vi "Checkers PvP.vi"() -> ()   [LabVIEW 2014]
uses:
  <vilib>/Utility/miscctls.llb/LVPositionTypeDef.ctl
  Game Info Global Variable.vi
  Board Layout Global Variable.vi
panel:
  out "P2 Piece 24":picture
  out "P2 Piece 23":picture
  out "P2 Piece 22":picture
  out "P2 Piece 21":picture
  out "P2 Piece 20":picture
  out "P2 Piece 19":picture
  out "P2 Piece 18":picture
  out "P2 Piece 17":picture
  out "P2 Piece 16":picture
  out "P2 Piece 15":picture
  out "P2 Piece 14":picture
  out "P2 Piece 13":picture
  out "P1 Piece 24":picture caption="P1 Piece"
  out "P1 Piece 23":picture caption="P1 Piece"
  out "P1 Piece 22":picture caption="P1 Piece"
  out "P1 Piece 21":picture caption="P1 Piece"
  out "P1 Piece 20":picture caption="P1 Piece"
  out "P1 Piece 19":picture caption="P1 Piece"
  out "P1 Piece 18":picture caption="P1 Piece"
  out "P1 Piece 17":picture caption="P1 Piece"
  out "P1 Piece 16":picture caption="P1 Piece"
  out "P1 Piece 15":picture caption="P1 Piece"
  out "P1 Piece 14":picture caption="P1 Piece"
  out "P1 Piece 13":picture caption="P1 Piece"
  out "P2 Bottom Right Marker":picture
  out "P2 Bottom Left Marker":picture
  out "P2 Top Left Marker":picture
  out "P2 Top Right Marker":picture
  out "P1 Bottom Left Marker":picture
  out "P1 Bottom Right Marker":picture
  out "P1 Top Right Marker":picture
  out "P1 Top Left Marker":picture
  in  "Save and Quit":bool
  out "Player 2 Name":string="Player 2"
  out "Player 1 Name":string="Player 1"
  out "P2 King 12":picture
  out "P2 King 11":picture
  out "P2 King 10":picture
  out "P2 King 9":picture
  out "P2 King 8":picture
  out "P2 King 7":picture
  out "P2 King 6":picture
  out "P2 King 5":picture
  out "P2 King 4":picture
  out "P2 King 3":picture
  out "P2 King 2":picture
  out "P2 King":picture
  out "P1 King 12":picture
  out "P1 King 11":picture
  out "P1 King 10":picture
  out "P1 King 9":picture
  out "P1 King 8":picture
  out "P1 King 7":picture
  out "P1 King 6":picture
  out "P1 King 5":picture
  out "P1 King 4":picture
  out "P1 King 3":picture
  out "P1 King 2":picture
  out "P1 King":picture
  out "P2 Piece Icon":picture
  out "P1 Piece Icon":picture
  out "P2 Piece 12":picture
  out "P2 Piece 11":picture
  out "P2 Piece 10":picture
  out "P2 Piece 9":picture
  out "P2 Piece 8":picture
  out "P2 Piece 7":picture
  out "P2 Piece 6":picture
  out "P2 Piece 5":picture
  out "P2 Piece 4":picture
  out "P2 Piece 3":picture
  out "P2 Piece 2":picture
  out "P1 Piece 12":picture caption="P1 Piece"
  out "P1 Piece 11":picture caption="P1 Piece"
  out "P1 Piece 10":picture caption="P1 Piece"
  out "P1 Piece 9":picture caption="P1 Piece"
  out "P1 Piece 8":picture caption="P1 Piece"
  out "P1 Piece 7":picture caption="P1 Piece"
  out "P1 Piece 6":picture caption="P1 Piece"
  out "P1 Piece 5":picture caption="P1 Piece"
  out "P1 Piece 4":picture caption="P1 Piece"
  out "P1 Piece 3":picture caption="P1 Piece"
  out "P2 Piece":picture
  out "P1 Piece 2":picture caption="P1 Piece"
  in  "TURN":bool
  out "Game String":string
  out "P2 Turn Light":bool
  out "P1 Turn Light":bool=TRUE
  out "P1 Piece":picture
  in  "stop":bool
  in  "Offer Draw":bool
  in  "Surrender":bool
  out "Player 2 Label":string="Player 1"
  out "Player 1 Label":string="Player 1"
  in  "Save":bool
  in  "Quit":bool
  # "Your Turn!"
  # "Your Turn!"
  # "678, \n56"
  # "764, \n56"
  # "512, \n56"
  # "594, \n56"
  # "637, \n99"
  # "469, \n99"
  # "553, \n99"
  # "720, \n99"
  # "355, \n141"
  # "400, \n141"
  # "512, \n140"
  # "594, \n140"
  # "678, \n140"
  # "828, \n141"
  # "873, \n141"
  # "764, \n140"
  # "828, \n184"
  # "873, \n184"
  # "355, \n184"
  # "400, \n184"
  # "469, \n183"
  # "553, \n183"
  # "637, \n183"
  # "720, \n183"
  # "355, \n225"
  # "828, \n225"
  # "873, \n225"
  # "400, \n225"
  # "764, \n224"
  # "512, \n224"
  # "595, \n224"
  # "678, \n224"
  # "828, \n267"
  # "873, \n267"
  # "355, \n267"
  # "400, \n267"
  # "469, \n266"
  # "553, \n266"
  # "720, \n266"
  # "637, \n266"
  # "355, \n309"
  # "828, \n309"
  # "400, \n309"
  # "873, \n309"
  # "678, \n308"
  # "764, \n308"
  # "512, \n308"
  # "595, \n308"
  # "355, \n351"
  # "400, \n351"
  # "873, \n351"
  # "828, \n351"
  # "553, \n350"
  # "637, \n350"
  # "720, \n350"
  # "469,\n350"
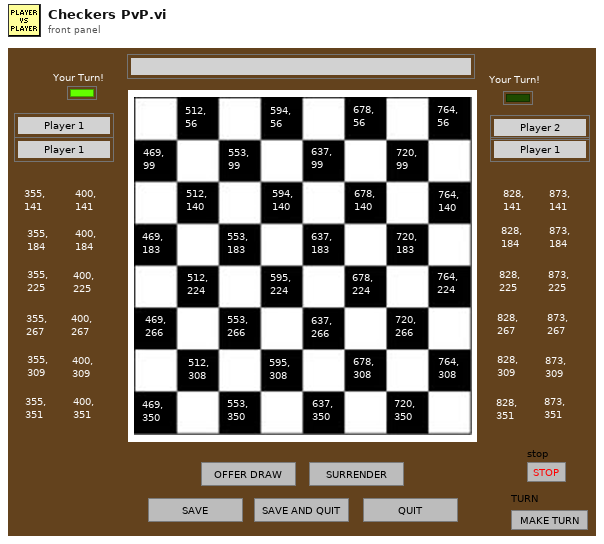
[diagram p1: front panel]
types:
  T1 = typedef "LVPositionTypeDef.ctl" = cluster{"Left":i32, "Top":i32}
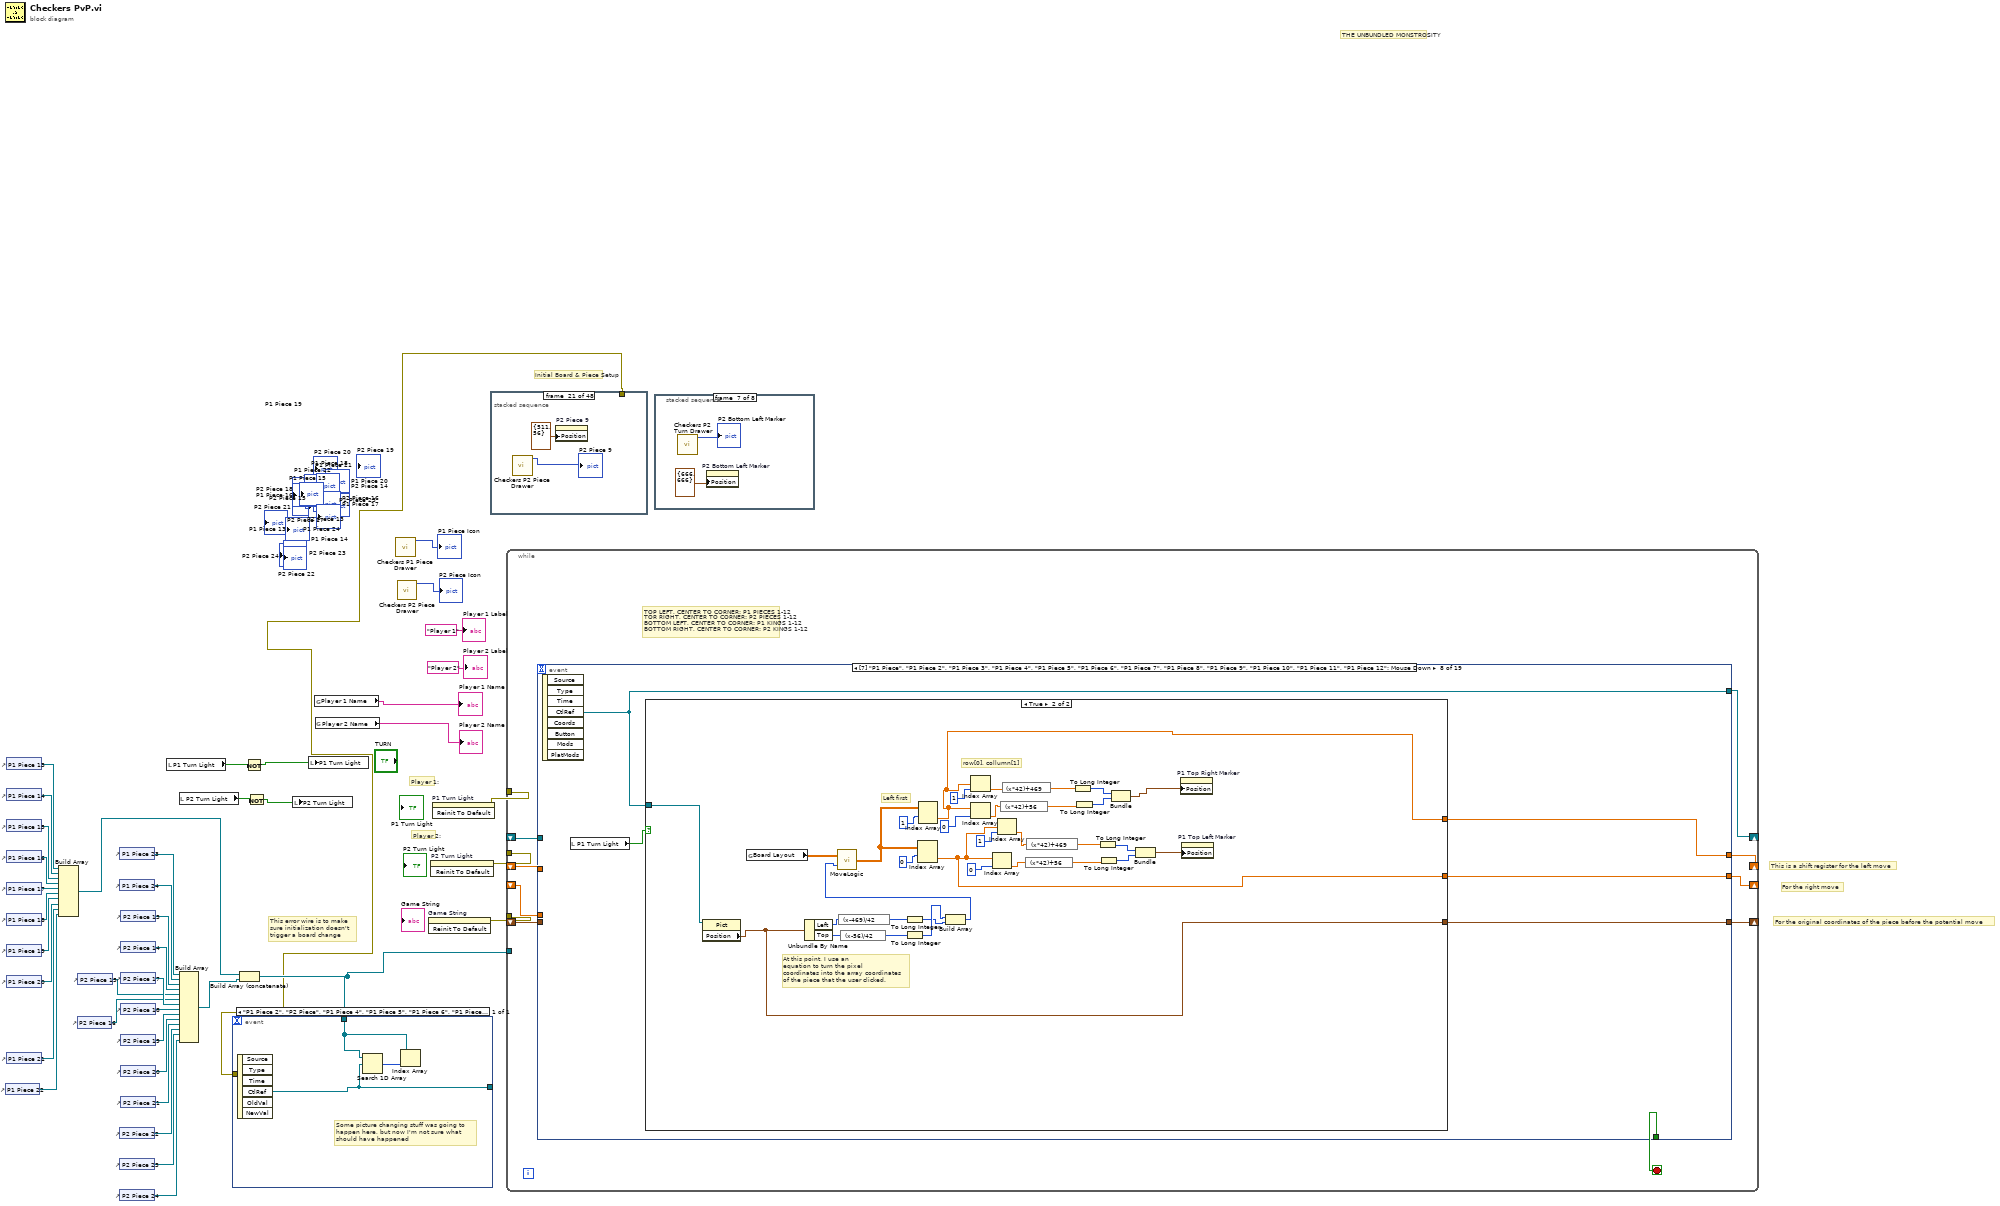
[diagram p0: block diagram]
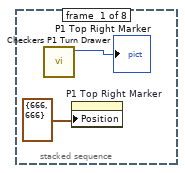
[diagram p2: hidden frame]
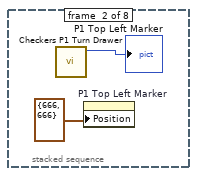
[diagram p3: hidden frame]
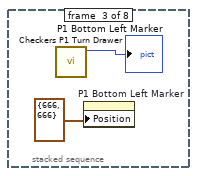
[diagram p4: hidden frame]
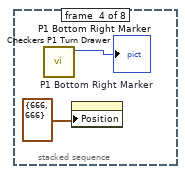
[diagram p5: hidden frame]
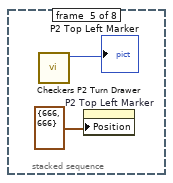
[diagram p6: hidden frame]
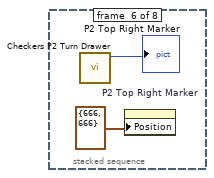
[diagram p7: hidden frame]
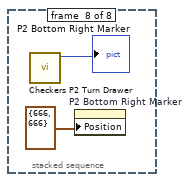
[diagram p8: hidden frame]
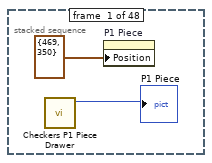
[diagram p9: hidden frame]
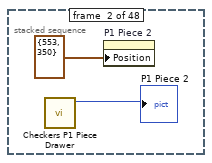
[diagram p10: hidden frame]
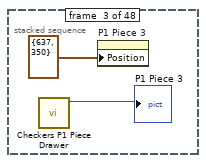
[diagram p11: hidden frame]
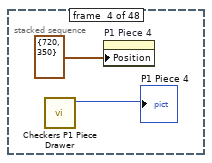
[diagram p12: hidden frame]
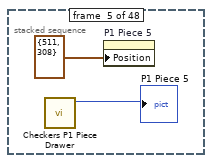
[diagram p13: hidden frame]
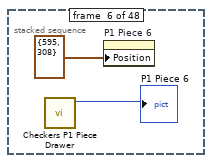
[diagram p14: hidden frame]
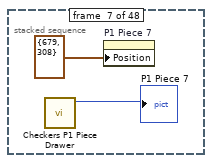
[diagram p15: hidden frame]
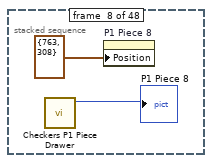
[diagram p16: hidden frame]
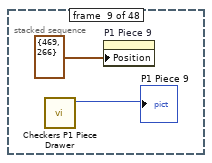
[diagram p17: hidden frame]
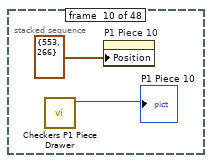
[diagram p18: hidden frame]
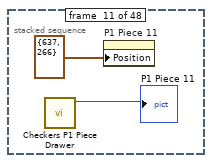
[diagram p19: hidden frame]
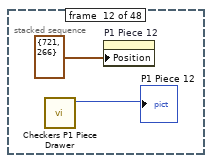
[diagram p20: hidden frame]
diagram:
  # "For the original coordinates of the piece before the potential move"
  # "For the right move"
  # "This error wire is to make \nsure initialization doesn't \ntrigger a board change"
  # "This is a shift register for the left move"
  # "THE UNBUNDLED MONSTROSITY"
  # "Initial Board & Piece Setup"
  # "Player 2:"
  # "Player 1:"
  n1 = control-ref of="P1 Piece 22"() -> (w104:refnum<vi>)
  n2 = control-ref of="P1 Piece 13"() -> (w113:refnum<vi>)
  n3 = control-ref of="P1 Piece 14"() -> (w112:refnum<vi>)
  n4 = control-ref of="P1 Piece 15"() -> (w111:refnum<vi>)
  n5 = control-ref of="P1 Piece 16"() -> (w110:refnum<vi>)
  n6 = control-ref of="P1 Piece 17"() -> (w109:refnum<vi>)
  n7 = control-ref of="P1 Piece 18"() -> (w108:refnum<vi>)
  n8 = control-ref of="P1 Piece 19"() -> (w107:refnum<vi>)
  n9 = control-ref of="P1 Piece 20"() -> (w106:refnum<vi>)
  n10 = control-ref of="P1 Piece 21"() -> (w105:refnum<vi>)
  n11 = Build Array(w113, w112, w111, w110, w109, w108, w107, w106, w105, w104) -> (w88:refnum<vi>[])
  n12 = control-ref of="P2 Piece 16"() -> (w95:refnum<vi>)
  n13 = control-ref of="P2 Piece 15"() -> (w96:refnum<vi>)
  n14 = control-ref of="P1 Piece 23"() -> (w103:refnum<vi>)
  n15 = control-ref of="P1 Piece 24"() -> (w102:refnum<vi>)
  n16 = control-ref of="P2 Piece 22"() -> (w92:refnum<vi>)
  n17 = control-ref of="P2 Piece 23"() -> (w91:refnum<vi>)
  n18 = control-ref of="P2 Piece 24"() -> (w90:refnum<vi>)
  n19 = control-ref of="P2 Piece 13"() -> (w101:refnum<vi>)
  n20 = control-ref of="P2 Piece 14"() -> (w100:refnum<vi>)
  n21 = control-ref of="P2 Piece 17"() -> (w99:refnum<vi>)
  n22 = control-ref of="P2 Piece 18"() -> (w98:refnum<vi>)
  n23 = control-ref of="P2 Piece 19"() -> (w97:refnum<vi>)
  n24 = control-ref of="P2 Piece 20"() -> (w94:refnum<vi>)
  n25 = control-ref of="P2 Piece 21"() -> (w93:refnum<vi>)
  n26 = local read "P1 Turn Light"() -> (w7:bool)
  n27 = local read "P1 Turn Light"() -> (w8:bool)
  n28 = local read "P1 Turn Light"() -> (w15:bool)
  n29 = local read "P1 Turn Light"() -> (w19:bool)
  n30 = local read "P1 Turn Light"() -> (w23:bool)
  n31 = local read "P1 Turn Light"() -> (w27:bool)
  n32 = local read "P1 Turn Light"() -> (w28:bool)
  n33 = local read "P1 Turn Light"() -> (w56:bool)
  n34 = local read "P1 Turn Light"() -> (w55:bool)
  n35 = local read "P1 Turn Light"() -> (w48:bool)
  n36 = local read "P1 Turn Light"() -> (w44:bool)
  n37 = local read "P1 Turn Light"() -> (w40:bool)
  n38 = local read "P1 Turn Light"() -> (w36:bool)
  n39 = local read "P1 Turn Light"() -> (w35:bool)
  n40 = local read "P1 Turn Light"() -> (w63:bool)
  n41 = local read "P1 Turn Light"() -> (w64:bool)
  n42 = local read "P1 Turn Light"() -> (w71:bool)
  n43 = local read "P1 Turn Light"() -> (w75:bool)
  n44 = local read "P1 Turn Light"() -> (w79:bool)
  n45 = local read "P1 Turn Light"() -> (w83:bool)
  n46 = local read "P1 Turn Light"() -> (w84:bool)
  n47 = local read "P2 Turn Light"() -> (w5:bool)
  n48 = local read "P2 Turn Light"() -> (w10:bool)
  n49 = local read "P2 Turn Light"() -> (w13:bool)
  n50 = local read "P2 Turn Light"() -> (w17:bool)
  n51 = local read "P2 Turn Light"() -> (w21:bool)
  n52 = local read "P2 Turn Light"() -> (w25:bool)
  n53 = local read "P2 Turn Light"() -> (w30:bool)
  n54 = local read "P2 Turn Light"() -> (w58:bool)
  n55 = local read "P2 Turn Light"() -> (w53:bool)
  n56 = local read "P2 Turn Light"() -> (w50:bool)
  n57 = local read "P2 Turn Light"() -> (w46:bool)
  n58 = local read "P2 Turn Light"() -> (w42:bool)
  n59 = local read "P2 Turn Light"() -> (w38:bool)
  n60 = local read "P2 Turn Light"() -> (w33:bool)
  n61 = local read "P2 Turn Light"() -> (w61:bool)
  n62 = local read "P2 Turn Light"() -> (w66:bool)
  n63 = local read "P2 Turn Light"() -> (w69:bool)
  n64 = local read "P2 Turn Light"() -> (w73:bool)
  n65 = local read "P2 Turn Light"() -> (w77:bool)
  n66 = local read "P2 Turn Light"() -> (w81:bool)
  n67 = local read "P2 Turn Light"() -> (w86:bool)
  n68 = Build Array(w103, w102, w101, w100, w96, w95, w99, w98, w97, w94, w93, w92, w91, w90) -> (w89:refnum<vi>[])
  n69 = Build Array (concatenate)(w88, w89) -> (w3:refnum<vi>[])
  n70 = Not(x=w7) -> (.not. x?=w6:bool)
  n71 = Not(x=w8) -> (.not. x?=w9:bool)
  n72 = Not(x=w15) -> (.not. x?=w14:bool)
  n73 = Not(x=w19) -> (.not. x?=w18:bool)
  n74 = Not(x=w23) -> (.not. x?=w22:bool)
  n75 = Not(x=w27) -> (.not. x?=w26:bool)
  n76 = Not(x=w28) -> (.not. x?=w29:bool)
  n77 = Not(x=w56) -> (.not. x?=w57:bool)
  n78 = Not(x=w55) -> (.not. x?=w54:bool)
  n79 = Not(x=w48) -> (.not. x?=w49:bool)
  n80 = Not(x=w44) -> (.not. x?=w45:bool)
  n81 = Not(x=w40) -> (.not. x?=w41:bool)
  n82 = Not(x=w36) -> (.not. x?=w37:bool)
  n83 = Not(x=w35) -> (.not. x?=w34:bool)
  n84 = Not(x=w63) -> (.not. x?=w62:bool)
  n85 = Not(x=w64) -> (.not. x?=w65:bool)
  n86 = Not(x=w71) -> (.not. x?=w70:bool)
  n87 = Not(x=w75) -> (.not. x?=w74:bool)
  n88 = Not(x=w79) -> (.not. x?=w78:bool)
  n89 = Not(x=w83) -> (.not. x?=w82:bool)
  n90 = Not(x=w84) -> (.not. x?=w85:bool)
  n91 = Not(x=w5) -> (.not. x?=w4:bool)
  n92 = Not(x=w10) -> (.not. x?=w11:bool)
  n93 = Not(x=w13) -> (.not. x?=w12:bool)
  n94 = Not(x=w17) -> (.not. x?=w16:bool)
  n95 = Not(x=w21) -> (.not. x?=w20:bool)
  n96 = Not(x=w25) -> (.not. x?=w24:bool)
  n97 = Not(x=w30) -> (.not. x?=w31:bool)
  n98 = Not(x=w58) -> (.not. x?=w59:bool)
  n99 = Not(x=w53) -> (.not. x?=w52:bool)
  n100 = Not(x=w50) -> (.not. x?=w51:bool)
  n101 = Not(x=w46) -> (.not. x?=w47:bool)
  n102 = Not(x=w42) -> (.not. x?=w43:bool)
  n103 = Not(x=w38) -> (.not. x?=w39:bool)
  n104 = Not(x=w33) -> (.not. x?=w32:bool)
  n105 = Not(x=w61) -> (.not. x?=w60:bool)
  n106 = Not(x=w66) -> (.not. x?=w67:bool)
  n107 = Not(x=w69) -> (.not. x?=w68:bool)
  n108 = Not(x=w73) -> (.not. x?=w72:bool)
  n109 = Not(x=w77) -> (.not. x?=w76:bool)
  n110 = Not(x=w81) -> (.not. x?=w80:bool)
  n111 = Not(x=w86) -> (.not. x?=w87:bool)
  n112 = local write "P2 Turn Light"(w4) -> ()
  n113 = local write "P2 Turn Light"(w11) -> ()
  n114 = local write "P2 Turn Light"(w12) -> ()
  n115 = local write "P2 Turn Light"(w16) -> ()
  n116 = local write "P2 Turn Light"(w20) -> ()
  n117 = local write "P2 Turn Light"(w24) -> ()
  n118 = local write "P2 Turn Light"(w31) -> ()
  n119 = local write "P2 Turn Light"(w59) -> ()
  n120 = local write "P2 Turn Light"(w52) -> ()
  n121 = local write "P2 Turn Light"(w51) -> ()
  n122 = local write "P2 Turn Light"(w47) -> ()
  n123 = local write "P2 Turn Light"(w43) -> ()
  n124 = local write "P2 Turn Light"(w39) -> ()
  n125 = local write "P2 Turn Light"(w32) -> ()
  n126 = local write "P2 Turn Light"(w60) -> ()
  n127 = local write "P2 Turn Light"(w67) -> ()
  n128 = local write "P2 Turn Light"(w68) -> ()
  n129 = local write "P2 Turn Light"(w72) -> ()
  n130 = local write "P2 Turn Light"(w76) -> ()
  n131 = local write "P2 Turn Light"(w80) -> ()
  n132 = local write "P2 Turn Light"(w87) -> ()
  n133 = local write "P1 Turn Light"(w6) -> ()
  n134 = local write "P1 Turn Light"(w9) -> ()
  n135 = local write "P1 Turn Light"(w14) -> ()
  n136 = local write "P1 Turn Light"(w18) -> ()
  n137 = local write "P1 Turn Light"(w22) -> ()
  n138 = local write "P1 Turn Light"(w26) -> ()
  n139 = local write "P1 Turn Light"(w29) -> ()
  n140 = local write "P1 Turn Light"(w57) -> ()
  n141 = local write "P1 Turn Light"(w54) -> ()
  n142 = local write "P1 Turn Light"(w49) -> ()
  n143 = local write "P1 Turn Light"(w45) -> ()
  n144 = local write "P1 Turn Light"(w41) -> ()
  n145 = local write "P1 Turn Light"(w37) -> ()
  n146 = local write "P1 Turn Light"(w34) -> ()
  n147 = local write "P1 Turn Light"(w62) -> ()
  n148 = local write "P1 Turn Light"(w65) -> ()
  n149 = local write "P1 Turn Light"(w70) -> ()
  n150 = local write "P1 Turn Light"(w74) -> ()
  n151 = local write "P1 Turn Light"(w78) -> ()
  n152 = local write "P1 Turn Light"(w82) -> ()
  n153 = local write "P1 Turn Light"(w85) -> ()
  n154 = global read "Game Info Global Variable.vi" "Player 1 Name"() -> (→"Player 1 Name":string)
  n155 = global read "Game Info Global Variable.vi" "Player 2 Name"() -> (→"Player 2 Name":string)
  n156 = call "Checkers P1 Piece Drawer.vi"() -> ("new picture"=→"P1 Piece Icon":picture)  [unwired: 11 in]
  n157 = call "Checkers P2 Piece Drawer.vi"() -> ("new picture"=→"P2 Piece Icon":picture)  [unwired: 11 in]
  n158 = invoke on="Game String" class="Str" method="Reinit To Default"() -> (error out=w117:errorcluster)  [unwired: 3 in, 2 out]
  n159 = invoke on="P2 Turn Light" class="Bool (strict)" method="Reinit To Default"() -> (error out=w119:errorcluster)  [unwired: 3 in, 2 out]
  n160 = invoke on="P1 Turn Light" class="Bool (strict)" method="Reinit To Default"() -> (error out=w118:errorcluster)  [unwired: 3 in, 2 out]
  n161 = stacked-sequence {
    tunnel: [_ _ _ _ _ _ _ _ _ _ _ _ _ _ _ _ _ _ _ _ _ _ _ _ _ _ _ _ _ _ _ _ _ _ _ _ _ _ _ _ _ _ _ _ _ _ _ w216] -> w1
    frame #0 {
      n162 = call "Checkers P1 Piece Drawer.vi"() -> ("new picture"=→"P1 Piece":picture)  [unwired: 11 in]
      n163 = property on="P1 Piece" class="Pict"("Position"=T1 {"Left"=469, "Top"=350}) -> ()  [unwired: 2 in, 2 out]
    }
    frame #1 {
      n164 = call "Checkers P1 Piece Drawer.vi"() -> ("new picture"=→"P1 Piece 2":picture)  [unwired: 11 in]
      n165 = property on="P1 Piece 2" class="Pict"("Position"=T1 {"Left"=553, "Top"=350}) -> ()  [unwired: 2 in, 2 out]
    }
    frame #2 {
      n166 = call "Checkers P1 Piece Drawer.vi"() -> ("new picture"=→"P1 Piece 3":picture)  [unwired: 11 in]
      n167 = property on="P1 Piece 3" class="Pict"("Position"=T1 {"Left"=637, "Top"=350}) -> ()  [unwired: 2 in, 2 out]
    }
    frame #3 {
      n168 = call "Checkers P1 Piece Drawer.vi"() -> ("new picture"=→"P1 Piece 4":picture)  [unwired: 11 in]
      n169 = property on="P1 Piece 4" class="Pict"("Position"=T1 {"Left"=720, "Top"=350}) -> ()  [unwired: 2 in, 2 out]
    }
    frame #4 {
      n170 = call "Checkers P1 Piece Drawer.vi"() -> ("new picture"=→"P1 Piece 5":picture)  [unwired: 11 in]
      n171 = property on="P1 Piece 5" class="Pict"("Position"=T1 {"Left"=511, "Top"=308}) -> ()  [unwired: 2 in, 2 out]
    }
    frame #5 {
      n172 = call "Checkers P1 Piece Drawer.vi"() -> ("new picture"=→"P1 Piece 6":picture)  [unwired: 11 in]
      n173 = property on="P1 Piece 6" class="Pict"("Position"=T1 {"Left"=595, "Top"=308}) -> ()  [unwired: 2 in, 2 out]
    }
    frame #6 {
      n174 = call "Checkers P1 Piece Drawer.vi"() -> ("new picture"=→"P1 Piece 7":picture)  [unwired: 11 in]
      n175 = property on="P1 Piece 7" class="Pict"("Position"=T1 {"Left"=679, "Top"=308}) -> ()  [unwired: 2 in, 2 out]
    }
    frame #7 {
      n176 = call "Checkers P1 Piece Drawer.vi"() -> ("new picture"=→"P1 Piece 8":picture)  [unwired: 11 in]
      n177 = property on="P1 Piece 8" class="Pict"("Position"=T1 {"Left"=763, "Top"=308}) -> ()  [unwired: 2 in, 2 out]
    }
    frame #8 {
      n178 = call "Checkers P1 Piece Drawer.vi"() -> ("new picture"=→"P1 Piece 9":picture)  [unwired: 11 in]
      n179 = property on="P1 Piece 9" class="Pict"("Position"=T1 {"Left"=469, "Top"=266}) -> ()  [unwired: 2 in, 2 out]
    }
    frame #9 {
      n180 = call "Checkers P1 Piece Drawer.vi"() -> ("new picture"=→"P1 Piece 10":picture)  [unwired: 11 in]
      n181 = property on="P1 Piece 10" class="Pict"("Position"=T1 {"Left"=553, "Top"=266}) -> ()  [unwired: 2 in, 2 out]
    }
    frame #10 {
      n182 = call "Checkers P1 Piece Drawer.vi"() -> ("new picture"=→"P1 Piece 11":picture)  [unwired: 11 in]
      n183 = property on="P1 Piece 11" class="Pict"("Position"=T1 {"Left"=637, "Top"=266}) -> ()  [unwired: 2 in, 2 out]
    }
    frame #11 {
      n184 = call "Checkers P1 Piece Drawer.vi"() -> ("new picture"=→"P1 Piece 12":picture)  [unwired: 11 in]
      n185 = property on="P1 Piece 12" class="Pict"("Position"=T1 {"Left"=721, "Top"=266}) -> ()  [unwired: 2 in, 2 out]
    }
    frame #12 {
      n186 = call "Checkers P2 Piece Drawer.vi"() -> ("new picture"=→"P2 Piece":picture)  [unwired: 11 in]
      n187 = property on="P2 Piece" class="Pict"("Position"=T1 {"Left"=511, "Top"=140}) -> ()  [unwired: 2 in, 2 out]
    }
    frame #13 {
      n188 = call "Checkers P2 Piece Drawer.vi"() -> ("new picture"=→"P2 Piece 2":picture)  [unwired: 11 in]
      n189 = property on="P2 Piece 2" class="Pict"("Position"=T1 {"Left"=595, "Top"=140}) -> ()  [unwired: 2 in, 2 out]
    }
    frame #14 {
      n190 = call "Checkers P2 Piece Drawer.vi"() -> ("new picture"=→"P2 Piece 3":picture)  [unwired: 11 in]
      n191 = property on="P2 Piece 3" class="Pict"("Position"=T1 {"Left"=679, "Top"=140}) -> ()  [unwired: 2 in, 2 out]
    }
    frame #15 {
      n192 = call "Checkers P2 Piece Drawer.vi"() -> ("new picture"=→"P2 Piece 4":picture)  [unwired: 11 in]
      n193 = property on="P2 Piece 4" class="Pict"("Position"=T1 {"Left"=763, "Top"=140}) -> ()  [unwired: 2 in, 2 out]
    }
    frame #16 {
      n194 = call "Checkers P2 Piece Drawer.vi"() -> ("new picture"=→"P2 Piece 5":picture)  [unwired: 11 in]
      n195 = property on="P2 Piece 5" class="Pict"("Position"=T1 {"Left"=469, "Top"=98}) -> ()  [unwired: 2 in, 2 out]
    }
    frame #17 {
      n196 = call "Checkers P2 Piece Drawer.vi"() -> ("new picture"=→"P2 Piece 6":picture)  [unwired: 11 in]
      n197 = property on="P2 Piece 6" class="Pict"("Position"=T1 {"Left"=553, "Top"=98}) -> ()  [unwired: 2 in, 2 out]
    }
    frame #18 {
      n198 = call "Checkers P2 Piece Drawer.vi"() -> ("new picture"=→"P2 Piece 7":picture)  [unwired: 11 in]
      n199 = property on="P2 Piece 7" class="Pict"("Position"=T1 {"Left"=637, "Top"=98}) -> ()  [unwired: 2 in, 2 out]
    }
    frame #19 {
      n200 = call "Checkers P2 Piece Drawer.vi"() -> ("new picture"=→"P2 Piece 8":picture)  [unwired: 11 in]
      n201 = property on="P2 Piece 8" class="Pict"("Position"=T1 {"Left"=721, "Top"=98}) -> ()  [unwired: 2 in, 2 out]
    }
    frame #20 {
      n202 = call "Checkers P2 Piece Drawer.vi"() -> ("new picture"=→"P2 Piece 9":picture)  [unwired: 11 in]
      n203 = property on="P2 Piece 9" class="Pict"("Position"=T1 {"Left"=511, "Top"=56}) -> ()  [unwired: 2 in, 2 out]
    }
    frame #21 {
      n204 = call "Checkers P2 Piece Drawer.vi"() -> ("new picture"=→"P2 Piece 10":picture)  [unwired: 11 in]
      n205 = property on="P2 Piece 10" class="Pict"("Position"=T1 {"Left"=595, "Top"=56}) -> ()  [unwired: 2 in, 2 out]
    }
    frame #22 {
      n206 = call "Checkers P2 Piece Drawer.vi"() -> ("new picture"=→"P2 Piece 11":picture)  [unwired: 11 in]
      n207 = property on="P2 Piece 11" class="Pict"("Position"=T1 {"Left"=679, "Top"=56}) -> ()  [unwired: 2 in, 2 out]
    }
    frame #23 {
      n208 = call "Checkers P2 Piece Drawer.vi"() -> ("new picture"=→"P2 Piece 12":picture)  [unwired: 11 in]
      n209 = property on="P2 Piece 12" class="Pict"("Position"=T1 {"Left"=763, "Top"=56}) -> ()  [unwired: 2 in, 2 out]
    }
    frame #24 {
      n210 = call "Checkers P1 King Drawer.vi"() -> ("new picture"=→"P1 King":picture)  [unwired: 11 in]
      n211 = property on="P1 King" class="Pict"("Position"=T1 {"Left"=666, "Top"=666}) -> ()  [unwired: 2 in, 2 out]
    }
    frame #25 {
      n212 = call "Checkers P1 King Drawer.vi"() -> ("new picture"=→"P1 King 2":picture)  [unwired: 11 in]
      n213 = property on="P1 King 2" class="Pict"("Position"=T1 {"Left"=666, "Top"=666}) -> ()  [unwired: 2 in, 2 out]
    }
    frame #26 {
      n214 = call "Checkers P1 King Drawer.vi"() -> ("new picture"=→"P1 King 3":picture)  [unwired: 11 in]
      n215 = property on="P1 King 3" class="Pict"("Position"=T1 {"Left"=666, "Top"=666}) -> ()  [unwired: 2 in, 2 out]
    }
    frame #27 {
      n216 = call "Checkers P1 King Drawer.vi"() -> ("new picture"=→"P1 King 4":picture)  [unwired: 11 in]
      n217 = property on="P1 King 4" class="Pict"("Position"=T1 {"Left"=666, "Top"=666}) -> ()  [unwired: 2 in, 2 out]
    }
    frame #28 {
      n218 = call "Checkers P1 King Drawer.vi"() -> ("new picture"=→"P1 King 5":picture)  [unwired: 11 in]
      n219 = property on="P1 King 5" class="Pict"("Position"=T1 {"Left"=666, "Top"=666}) -> ()  [unwired: 2 in, 2 out]
    }
    frame #29 {
      n220 = call "Checkers P1 King Drawer.vi"() -> ("new picture"=→"P1 King 6":picture)  [unwired: 11 in]
      n221 = property on="P1 King 6" class="Pict"("Position"=T1 {"Left"=666, "Top"=666}) -> ()  [unwired: 2 in, 2 out]
    }
    frame #30 {
      n222 = call "Checkers P1 King Drawer.vi"() -> ("new picture"=→"P1 King 7":picture)  [unwired: 11 in]
      n223 = property on="P1 King 7" class="Pict"("Position"=T1 {"Left"=666, "Top"=666}) -> ()  [unwired: 2 in, 2 out]
    }
    frame #31 {
      n224 = call "Checkers P1 King Drawer.vi"() -> ("new picture"=→"P1 King 8":picture)  [unwired: 11 in]
      n225 = property on="P1 King 8" class="Pict"("Position"=T1 {"Left"=666, "Top"=666}) -> ()  [unwired: 2 in, 2 out]
    }
    frame #32 {
      n226 = call "Checkers P1 King Drawer.vi"() -> ("new picture"=→"P1 King 9":picture)  [unwired: 11 in]
      n227 = property on="P1 King 9" class="Pict"("Position"=T1 {"Left"=666, "Top"=666}) -> ()  [unwired: 2 in, 2 out]
    }
    frame #33 {
      n228 = call "Checkers P1 King Drawer.vi"() -> ("new picture"=→"P1 King 10":picture)  [unwired: 11 in]
      n229 = property on="P1 King 10" class="Pict"("Position"=T1 {"Left"=666, "Top"=666}) -> ()  [unwired: 2 in, 2 out]
    }
    frame #34 {
      n230 = call "Checkers P1 King Drawer.vi"() -> ("new picture"=→"P1 King 11":picture)  [unwired: 11 in]
      n231 = property on="P1 King 11" class="Pict"("Position"=T1 {"Left"=666, "Top"=666}) -> ()  [unwired: 2 in, 2 out]
    }
    frame #35 {
      n232 = call "Checkers P1 King Drawer.vi"() -> ("new picture"=→"P1 King 12":picture)  [unwired: 11 in]
      n233 = property on="P1 King 12" class="Pict"("Position"=T1 {"Left"=666, "Top"=666}) -> ()  [unwired: 2 in, 2 out]
    }
    frame #36 {
      n234 = call "Checkers P2 King Drawer.vi"() -> ("new picture"=→"P2 King":picture)  [unwired: 11 in]
      n235 = property on="P2 King" class="Pict"("Position"=T1 {"Left"=666, "Top"=666}) -> ()  [unwired: 2 in, 2 out]
    }
    frame #37 {
      n236 = call "Checkers P2 King Drawer.vi"() -> ("new picture"=→"P2 King 2":picture)  [unwired: 11 in]
      n237 = property on="P2 King 2" class="Pict"("Position"=T1 {"Left"=666, "Top"=666}) -> ()  [unwired: 2 in, 2 out]
    }
    frame #38 {
      n238 = call "Checkers P2 King Drawer.vi"() -> ("new picture"=→"P2 King 3":picture)  [unwired: 11 in]
      n239 = property on="P2 King 3" class="Pict"("Position"=T1 {"Left"=666, "Top"=666}) -> ()  [unwired: 2 in, 2 out]
    }
    frame #39 {
      n240 = call "Checkers P2 King Drawer.vi"() -> ("new picture"=→"P2 King 4":picture)  [unwired: 11 in]
      n241 = property on="P2 King 4" class="Pict"("Position"=T1 {"Left"=666, "Top"=666}) -> ()  [unwired: 2 in, 2 out]
    }
    frame #40 {
      n242 = call "Checkers P2 King Drawer.vi"() -> ("new picture"=→"P2 King 5":picture)  [unwired: 11 in]
      n243 = property on="P2 King 5" class="Pict"("Position"=T1 {"Left"=666, "Top"=666}) -> ()  [unwired: 2 in, 2 out]
    }
    frame #41 {
      n244 = call "Checkers P2 King Drawer.vi"() -> ("new picture"=→"P2 King 6":picture)  [unwired: 11 in]
      n245 = property on="P2 King 6" class="Pict"("Position"=T1 {"Left"=666, "Top"=666}) -> ()  [unwired: 2 in, 2 out]
    }
    frame #42 {
      n246 = call "Checkers P2 King Drawer.vi"() -> ("new picture"=→"P2 King 7":picture)  [unwired: 11 in]
      n247 = property on="P2 King 7" class="Pict"("Position"=T1 {"Left"=666, "Top"=666}) -> ()  [unwired: 2 in, 2 out]
    }
    frame #43 {
      n248 = call "Checkers P2 King Drawer.vi"() -> ("new picture"=→"P2 King 8":picture)  [unwired: 11 in]
      n249 = property on="P2 King 8" class="Pict"("Position"=T1 {"Left"=666, "Top"=666}) -> ()  [unwired: 2 in, 2 out]
    }
    frame #44 {
      n250 = call "Checkers P2 King Drawer.vi"() -> ("new picture"=→"P2 King 9":picture)  [unwired: 11 in]
      n251 = property on="P2 King 9" class="Pict"("Position"=T1 {"Left"=666, "Top"=666}) -> ()  [unwired: 2 in, 2 out]
    }
    frame #45 {
      n252 = call "Checkers P2 King Drawer.vi"() -> ("new picture"=→"P2 King 10":picture)  [unwired: 11 in]
      n253 = property on="P2 King 10" class="Pict"("Position"=T1 {"Left"=666, "Top"=666}) -> ()  [unwired: 2 in, 2 out]
    }
    frame #46 {
      n254 = call "Checkers P2 King Drawer.vi"() -> ("new picture"=→"P2 King 11":picture)  [unwired: 11 in]
      n255 = property on="P2 King 11" class="Pict"("Position"=T1 {"Left"=666, "Top"=666}) -> ()  [unwired: 2 in, 2 out]
    }
    frame #47 {
      n256 = call "Checkers P2 King Drawer.vi"() -> ("new picture"=→"P2 King 12":picture)  [unwired: 11 in]
      n257 = property on="P2 King 12" class="Pict"("Position"=T1 {"Left"=666, "Top"=666}) -> (error out=w216:errorcluster)  [unwired: 2 in, 1 out]
    }
  }
  n258 = event shown="[0] \"P1 Piece 2\", \"P2 Piece\", \"P1 Piece 4\", \"P1 Piece 5\", \"P1 Piece 6\", \"P1 Piece 7\", \"P1 Piece 8\", \"P1 Piece 9\", \"P1 Piece 10\", \"P1 Piece 11\", \"P1 Piece 12\", \"P2 Piece 2\", \"P2 Piece 3\", \"P2 Piece 4\", \"P2 Piece 6\", \"P2 Piece 7\", \"P2 Piece 8\", \"P2 Piece 9\", \"P2 Piece 10\", \"P2 Piece 11\", \"P2 Piece 12\": Value Change" {
    selector: _ -> [_]
    dyn-events: _ -> [_]
    timeout: _ -> [_]
    tunnel: [w221] -> _
    tunnel: w3 -> [w220]
    tunnel: w1 -> [_]
    event "P1 Piece 2", "P2 Piece", "P1 Piece 4", "P1 Piece 5", "P1 Piece 6", "P1 Piece 7", "P1 Piece 8", "P1 Piece 9", "P1 Piece 10", "P1 Piece 11", "P1 Piece 12", "P2 Piece 2", "P2 Piece 3", "P2 Piece 4", "P2 Piece 6", "P2 Piece 7", "P2 Piece 8", "P2 Piece 9", "P2 Piece 10", "P2 Piece 11", "P2 Piece 12": Value Change {
      # "Some picture changing stuff was going to \nhappen here, but now I'm not sure what \nshould have happened"
      n259 = event-data() -> ("CtlRef"=w221:refnum<vi>)  [unwired: 1 in, 5 out]
      n260 = Search 1D Array(1D array=w220, element=w221) -> (index of element=w219:i32)  [unwired: 1 in]
      n261 = Index Array(array=w220, index=w219) -> ()  [unwired: 1 out]
    }
  }
  n262 = while {
    tunnel: w119 -> [_]
    tunnel: w118 -> [_]
    tunnel: w117 -> [_]
    tunnel: w3 -> [_]
    shift-right: [w229] -> _
    shift-left: _ -> [w228]
    shift-right: [w227] -> _
    shift-left: _ -> [w222]
    shift-right: [w226] -> _
    shift-left: _ -> [w225]
    shift-right: [w224] -> _
    shift-left: _ -> [w223]
    stop <- w230 stop-if-true
    # "TOP LEFT, CENTER TO CORNER: P1 PIECES 1-12\nTOR RIGHT, CENTER TO CORNER: P2 PIECES 1-12\nBOTTOM LEFT, CENTER TO CORNER: P1 KINGS 1-12\nBOTTOM RIGHT, CENTER TO CORNER: P2 KINGS 1-12"
    n263 = event shown="[7] \"P1 Piece\", \"P1 Piece 2\", \"P1 Piece 3\", \"P1 Piece 4\", \"P1 Piece 5\", \"P1 Piece 6\", \"P1 Piece 7\", \"P1 Piece 8\", \"P1 Piece 9\", \"P1 Piece 10\", \"P1 Piece 11\", \"P1 Piece 12\": Mouse Down" {
      selector: _ -> [_ _ _ _ _ _ _ _ _ _ _ _ _ _ _ _ _ _ _]
      dyn-events: _ -> [_ _ _ _ _ _ _ _ _ _ _ _ _ _ _ _ _ _ _]
      timeout: _ -> [_ _ _ _ _ _ _ _ _ _ _ _ _ _ _ _ _ _ _]
      tunnel: [_ "stop" _ _ _ _ _ _ _ _ _ _ _ _ _ _ _ _ _] -> w230
      tunnel: [_ _ _ _ _ _ _ w605 w640 w675 w710 _ _ _ _ _ _ _ _] -> w229
      tunnel: w228 -> [_ _ _ _ _ _ _ _ _ _ _ w755 w766 w777 w788 w799 w814 w849 w940]
      tunnel: [_ _ _ _ _ _ _ w604 _ _ _ _ _ _ _ _ _ _ _] -> w227
      tunnel: [_ _ _ _ _ _ _ w603 _ _ _ _ _ _ _ _ _ _ _] -> w226
      tunnel: w225 -> [_ _ _ _ _ _ _ _ _ _ _ w748 _ _ _ _ _ _ _]
      tunnel: [_ _ _ _ _ _ _ w602 _ _ _ _ _ _ _ _ _ _ _] -> w224
      tunnel: w223 -> [_ _ _ _ _ _ _ _ _ _ _ w747 _ _ _ _ w801 _ _]
      tunnel: w222 -> [_ _ _ _ _ _ _ _ _ _ _ _ _ _ _ _ w800 _ _]
      event Timeout {
        n264 = event-data() -> ()  [unwired: 1 in, 3 out]
      }
      event "stop": Value Change {
        n265 = event-data() -> ()  [unwired: 1 in, 6 out]
      }
      event "Offer Draw": Value Change {
        n266 = event-data() -> ()  [unwired: 1 in, 6 out]
        n267 = local read "P1 Turn Light"() -> (w232:bool)
        n268 = case shown="False" w232 {
          frame False {
            n269 = local read "Player 2 Name"() -> (w236:string)
            n270 = Format Into String(format string="%s offers a stalemate. Do you accept?", w236) -> (resulting string=w234:string)  [unwired: 2 in, 1 out]
            n271 = Two Button Dialog(message=w234, 1:"Decline" ("F button name (\"Cancel\")"), 2:"Accept" ("T button name (\"OK\")")) -> (T button?=w233:bool)
            n272 = case shown="True" w233 {
              frame False {
                # "Stalemate offer rejected. Do nothing."
              }
              frame True {
                w239 = "GAME OVER. It's a draw." ("format string")
                n273 = local write "Game String"(w239) -> ()
                n274 = Two Button Dialog(message=w239, 1:"Main Menu" ("F button name (\"Cancel\")"), 2:"New Game" ("T button name (\"OK\")")) -> (T button?=w242:bool)
                n275 = case shown="False" w242 {
                  frame False {
                    n276 = vi-ref "Checkers Main Menu.vi"() -> (w249:refnum<vi>)
                    n277 = invoke class="VI" method="Run VI"(reference=w249, "Wait until done"=FALSE ("Wait Until Done")) -> (reference out=w248:refnum<vi>, error out=w247:errorcluster)  [unwired: 3 in, 3 out]
                    n278 = invoke class="VI" method="FP.Open"(reference=w248, error in=w247, "Activate"=TRUE ("Activate?")) -> (error out=w246:errorcluster)  [unwired: 2 in, 4 out]
                    n279 = vi-ref "Checkers PvP.vi"() -> (w245:refnum<vi>)
                    n280 = invoke class="VI" method="Abort VI"(reference=w245, error in=w246) -> ()  [unwired: 1 in, 3 out]
                  }
                  frame True {
                    n281 = vi-ref "Checkers New Game.vi"() -> (w256:refnum<vi>)
                    n282 = invoke class="VI" method="Run VI"(reference=w256, "Wait until done"=FALSE ("Wait Until Done")) -> (reference out=w255:refnum<vi>, error out=w254:errorcluster)  [unwired: 3 in, 3 out]
                    n283 = invoke class="VI" method="FP.Open"(reference=w255, error in=w254, "Activate"=TRUE ("Activate?")) -> (error out=w253:errorcluster)  [unwired: 2 in, 4 out]
                    n284 = vi-ref "Checkers PvP.vi"() -> (w252:refnum<vi>)
                    n285 = invoke class="VI" method="Abort VI"(reference=w252, error in=w253) -> ()  [unwired: 1 in, 3 out]
                  }
                }
              }
            }
          }
          frame True {
            n286 = local read "Player 1 Name"() -> (w260:string)
            n287 = Format Into String(format string="%s offers a stalemate. Do you accept?", w260) -> (resulting string=w258:string)  [unwired: 2 in, 1 out]
            n288 = Two Button Dialog(message=w258, 1:"Decline" ("F button name (\"Cancel\")"), 2:"Accept" ("T button name (\"OK\")")) -> (T button?=w257:bool)
            n289 = case shown="True" w257 {
              frame False {
                # "Stalemate offer was rejected. Do nothing."
              }
              frame True {
                w263 = "GAME OVER. Stalemate." ("format string")
                n290 = local write "Game String"(w263) -> ()
                n291 = Two Button Dialog(message=w263, 1:"Main Menu" ("F button name (\"Cancel\")"), 2:"New Game" ("T button name (\"OK\")")) -> (T button?=w266:bool)
                n292 = case shown="False" w266 {
                  frame False {
                    n293 = vi-ref "Checkers Main Menu.vi"() -> (w273:refnum<vi>)
                    n294 = invoke class="VI" method="Run VI"(reference=w273, "Wait until done"=FALSE ("Wait Until Done")) -> (reference out=w272:refnum<vi>, error out=w271:errorcluster)  [unwired: 3 in, 3 out]
                    n295 = invoke class="VI" method="FP.Open"(reference=w272, error in=w271, "Activate"=TRUE ("Activate?")) -> (error out=w270:errorcluster)  [unwired: 2 in, 4 out]
                    n296 = vi-ref "Checkers PvP.vi"() -> (w269:refnum<vi>)
                    n297 = invoke class="VI" method="Abort VI"(reference=w269, error in=w270) -> ()  [unwired: 1 in, 3 out]
                  }
                  frame True {
                    n298 = vi-ref "Checkers New Game.vi"() -> (w280:refnum<vi>)
                    n299 = invoke class="VI" method="Run VI"(reference=w280, "Wait until done"=FALSE ("Wait Until Done")) -> (reference out=w279:refnum<vi>, error out=w278:errorcluster)  [unwired: 3 in, 3 out]
                    n300 = invoke class="VI" method="FP.Open"(reference=w279, error in=w278, "Activate"=TRUE ("Activate?")) -> (error out=w277:errorcluster)  [unwired: 2 in, 4 out]
                    n301 = vi-ref "Checkers PvP.vi"() -> (w276:refnum<vi>)
                    n302 = invoke class="VI" method="Abort VI"(reference=w276, error in=w277) -> ()  [unwired: 1 in, 3 out]
                  }
                }
              }
            }
          }
        }
      }
      event "Surrender": Value Change {
        n303 = event-data() -> ()  [unwired: 1 in, 6 out]
        n304 = Two Button Dialog(message="Are you sure you want to surrender?", 1:"No" ("F button name (\"Cancel\")"), 2:"Yes" ("T button name (\"OK\")")) -> (T button?=w281:bool)
        n305 = case shown="True" w281 {
          frame False {
            # "Player changed mind, didn't surrender. Do nothing."
          }
          frame True {
            n306 = local read "P1 Turn Light"() -> (w285:bool)
            n307 = case shown="True" w285 {
              frame False {
                n308 = local read "Player 1 Name"() -> (w286:string)
                n309 = Format Into String(format string="GAME OVER. %s WINS!", w286) -> (resulting string=w290:string)  [unwired: 2 in, 1 out]
                n310 = local write "Game String"(w290) -> ()
                n311 = Two Button Dialog(message=w290, 1:"Main Menu" ("F button name (\"Cancel\")"), 2:"New Game" ("T button name (\"OK\")")) -> (T button?=w287:bool)
                n312 = case shown="True" w287 {
                  frame False {
                    n313 = vi-ref "Checkers Main Menu.vi"() -> (w298:refnum<vi>)
                    n314 = invoke class="VI" method="Run VI"(reference=w298, "Wait until done"=FALSE ("Wait Until Done")) -> (reference out=w297:refnum<vi>, error out=w296:errorcluster)  [unwired: 3 in, 3 out]
                    n315 = invoke class="VI" method="FP.Open"(reference=w297, error in=w296, "Activate"=TRUE ("Activate?")) -> (error out=w295:errorcluster)  [unwired: 2 in, 4 out]
                    n316 = vi-ref "Checkers PvP.vi"() -> (w294:refnum<vi>)
                    n317 = invoke class="VI" method="Abort VI"(reference=w294, error in=w295) -> ()  [unwired: 1 in, 3 out]
                  }
                  frame True {
                    n318 = vi-ref "Checkers New Game.vi"() -> (w308:refnum<vi>)
                    n319 = vi-ref "Checkers Gymnopedie Music Player.vi"() -> (w299:refnum<vi>)
                    n320 = invoke class="VI" method="Run VI"(reference=w299, "Wait until done"=FALSE ("Wait Until Done")) -> ()  [unwired: 3 in, 5 out]
                    n321 = invoke class="VI" method="Run VI"(reference=w308, "Wait until done"=FALSE ("Wait Until Done")) -> (reference out=w307:refnum<vi>, error out=w306:errorcluster)  [unwired: 3 in, 3 out]
                    n322 = vi-ref "Checkers Palladio Music Player.vi"() -> (w301:refnum<vi>)
                    n323 = invoke class="VI" method="FP.Open"(reference=w307, error in=w306, "Activate"=TRUE ("Activate?")) -> (error out=w305:errorcluster)  [unwired: 2 in, 4 out]
                    n324 = vi-ref "Checkers PvP.vi"() -> (w304:refnum<vi>)
                    n325 = invoke class="VI" method="Abort VI"(reference=w301) -> ()  [unwired: 2 in, 3 out]
                    n326 = invoke class="VI" method="Abort VI"(reference=w304, error in=w305) -> ()  [unwired: 1 in, 3 out]
                  }
                }
              }
              frame True {
                n327 = local read "Player 2 Name"() -> (w309:string)
                n328 = Format Into String(format string="GAME OVER. %s WINS!", w309) -> (resulting string=w313:string)  [unwired: 2 in, 1 out]
                n329 = local write "Game String"(w313) -> ()
                n330 = Two Button Dialog(message=w313, 1:"Main Menu" ("F button name (\"Cancel\")"), 2:"New Game" ("T button name (\"OK\")")) -> (T button?=w310:bool)
                n331 = case shown="True" w310 {
                  frame False {
                    n332 = vi-ref "Checkers Main Menu.vi"() -> (w321:refnum<vi>)
                    n333 = invoke class="VI" method="Run VI"(reference=w321, "Wait until done"=FALSE ("Wait Until Done")) -> (reference out=w320:refnum<vi>, error out=w319:errorcluster)  [unwired: 3 in, 3 out]
                    n334 = invoke class="VI" method="FP.Open"(reference=w320, error in=w319, "Activate"=TRUE ("Activate?")) -> (error out=w318:errorcluster)  [unwired: 2 in, 4 out]
                    n335 = vi-ref "Checkers PvP.vi"() -> (w317:refnum<vi>)
                    n336 = invoke class="VI" method="Abort VI"(reference=w317, error in=w318) -> ()  [unwired: 1 in, 3 out]
                  }
                  frame True {
                    n337 = vi-ref "Checkers New Game.vi"() -> (w331:refnum<vi>)
                    n338 = vi-ref "Checkers Gymnopedie Music Player.vi"() -> (w322:refnum<vi>)
                    n339 = invoke class="VI" method="Run VI"(reference=w331, "Wait until done"=FALSE ("Wait Until Done")) -> (reference out=w330:refnum<vi>, error out=w329:errorcluster)  [unwired: 3 in, 3 out]
                    n340 = invoke class="VI" method="Run VI"(reference=w322, "Wait until done"=FALSE ("Wait Until Done")) -> ()  [unwired: 3 in, 5 out]
                    n341 = vi-ref "Checkers Palladio Music Player.vi"() -> (w324:refnum<vi>)
                    n342 = invoke class="VI" method="FP.Open"(reference=w330, error in=w329, "Activate"=TRUE ("Activate?")) -> (error out=w328:errorcluster)  [unwired: 2 in, 4 out]
                    n343 = vi-ref "Checkers PvP.vi"() -> (w327:refnum<vi>)
                    n344 = invoke class="VI" method="Abort VI"(reference=w324) -> ()  [unwired: 2 in, 3 out]
                    n345 = invoke class="VI" method="Abort VI"(reference=w327, error in=w328) -> ()  [unwired: 1 in, 3 out]
                  }
                }
              }
            }
          }
        }
      }
      event "Save": Value Change {
        n346 = event-data() -> ()  [unwired: 1 in, 6 out]
        n347 = global read "Game Info Global Variable.vi" "P1 King Text Green Color"() -> (w391:i32)
        n348 = global read "Game Info Global Variable.vi" "P2 King Text Green Color"() -> (w385:i32)
        n349 = global read "Game Info Global Variable.vi" "P1 King Text Blue Color"() -> (w390:i32)
        n350 = global read "Game Info Global Variable.vi" "P2 King Text Blue Color"() -> (w384:i32)
        n351 = global read "Game Info Global Variable.vi" "P1 King Text Red Color"() -> (w392:i32)
        n352 = global read "Game Info Global Variable.vi" "P2 King Text Red Color"() -> (w386:i32)
        n353 = global read "Game Info Global Variable.vi" "P1 Green Color"() -> (w394:i32)
        n354 = global read "Game Info Global Variable.vi" "P2 Green Color"() -> (w388:i32)
        n355 = local read "Player 1 Name"() -> (w398:string)
        n356 = local read "Player 2 Name"() -> (w397:string)
        n357 = global read "Game Info Global Variable.vi" "P1 Red Color"() -> (w395:i32)
        n358 = global read "Game Info Global Variable.vi" "P1 Blue Color"() -> (w393:i32)
        n359 = global read "Game Info Global Variable.vi" "P2 Blue Color"() -> (w387:i32)
        n360 = global read "Game Info Global Variable.vi" "P2 Red Color"() -> (w389:i32)
        n361 = Format Into String(w398, w397, w395, w394, w393, w392, w391, w390, w389, w388, w387, w386, w385, w384) -> (resulting string=w396:refnum<file>)  [unwired: 3 in, 1 out]
        n362 = stacked-sequence {
          tunnel: [w399 _ _ _ _ _ _ _ _ _ _ _ _ _ _ _ _ _ _ _ _ _ _ _ _ _ _ _ _ _ _ _ _ _ _ _ _ _ _ _ _ _ _ _ _ _ _ _] -> w383
          tunnel: [_ w400 _ _ _ _ _ _ _ _ _ _ _ _ _ _ _ _ _ _ _ _ _ _ _ _ _ _ _ _ _ _ _ _ _ _ _ _ _ _ _ _ _ _ _ _ _ _] -> w382
          tunnel: [_ _ w401 _ _ _ _ _ _ _ _ _ _ _ _ _ _ _ _ _ _ _ _ _ _ _ _ _ _ _ _ _ _ _ _ _ _ _ _ _ _ _ _ _ _ _ _ _] -> w381
          tunnel: [_ _ _ w402 _ _ _ _ _ _ _ _ _ _ _ _ _ _ _ _ _ _ _ _ _ _ _ _ _ _ _ _ _ _ _ _ _ _ _ _ _ _ _ _ _ _ _ _] -> w380
          tunnel: [_ _ _ _ w403 _ _ _ _ _ _ _ _ _ _ _ _ _ _ _ _ _ _ _ _ _ _ _ _ _ _ _ _ _ _ _ _ _ _ _ _ _ _ _ _ _ _ _] -> w379
          tunnel: [_ _ _ _ _ w404 _ _ _ _ _ _ _ _ _ _ _ _ _ _ _ _ _ _ _ _ _ _ _ _ _ _ _ _ _ _ _ _ _ _ _ _ _ _ _ _ _ _] -> w378
          tunnel: [_ _ _ _ _ _ w405 _ _ _ _ _ _ _ _ _ _ _ _ _ _ _ _ _ _ _ _ _ _ _ _ _ _ _ _ _ _ _ _ _ _ _ _ _ _ _ _ _] -> w377
          tunnel: [_ _ _ _ _ _ _ w406 _ _ _ _ _ _ _ _ _ _ _ _ _ _ _ _ _ _ _ _ _ _ _ _ _ _ _ _ _ _ _ _ _ _ _ _ _ _ _ _] -> w376
          tunnel: [_ _ _ _ _ _ _ _ w407 _ _ _ _ _ _ _ _ _ _ _ _ _ _ _ _ _ _ _ _ _ _ _ _ _ _ _ _ _ _ _ _ _ _ _ _ _ _ _] -> w375
          tunnel: [_ _ _ _ _ _ _ _ _ w408 _ _ _ _ _ _ _ _ _ _ _ _ _ _ _ _ _ _ _ _ _ _ _ _ _ _ _ _ _ _ _ _ _ _ _ _ _ _] -> w374
          tunnel: [_ _ _ _ _ _ _ _ _ _ w409 _ _ _ _ _ _ _ _ _ _ _ _ _ _ _ _ _ _ _ _ _ _ _ _ _ _ _ _ _ _ _ _ _ _ _ _ _] -> w373
          tunnel: [_ _ _ _ _ _ _ _ _ _ _ w410 _ _ _ _ _ _ _ _ _ _ _ _ _ _ _ _ _ _ _ _ _ _ _ _ _ _ _ _ _ _ _ _ _ _ _ _] -> w372
          tunnel: [_ _ _ _ _ _ _ _ _ _ _ _ w411 _ _ _ _ _ _ _ _ _ _ _ _ _ _ _ _ _ _ _ _ _ _ _ _ _ _ _ _ _ _ _ _ _ _ _] -> w370
          tunnel: [_ _ _ _ _ _ _ _ _ _ _ _ _ w412 _ _ _ _ _ _ _ _ _ _ _ _ _ _ _ _ _ _ _ _ _ _ _ _ _ _ _ _ _ _ _ _ _ _] -> w369
          tunnel: [_ _ _ _ _ _ _ _ _ _ _ _ _ _ w413 _ _ _ _ _ _ _ _ _ _ _ _ _ _ _ _ _ _ _ _ _ _ _ _ _ _ _ _ _ _ _ _ _] -> w368
          tunnel: [_ _ _ _ _ _ _ _ _ _ _ _ _ _ _ w414 _ _ _ _ _ _ _ _ _ _ _ _ _ _ _ _ _ _ _ _ _ _ _ _ _ _ _ _ _ _ _ _] -> w367
          tunnel: [_ _ _ _ _ _ _ _ _ _ _ _ _ _ _ _ w415 _ _ _ _ _ _ _ _ _ _ _ _ _ _ _ _ _ _ _ _ _ _ _ _ _ _ _ _ _ _ _] -> w366
          tunnel: [_ _ _ _ _ _ _ _ _ _ _ _ _ _ _ _ _ w416 _ _ _ _ _ _ _ _ _ _ _ _ _ _ _ _ _ _ _ _ _ _ _ _ _ _ _ _ _ _] -> w365
          tunnel: [_ _ _ _ _ _ _ _ _ _ _ _ _ _ _ _ _ _ w417 _ _ _ _ _ _ _ _ _ _ _ _ _ _ _ _ _ _ _ _ _ _ _ _ _ _ _ _ _] -> w364
          tunnel: [_ _ _ _ _ _ _ _ _ _ _ _ _ _ _ _ _ _ _ w418 _ _ _ _ _ _ _ _ _ _ _ _ _ _ _ _ _ _ _ _ _ _ _ _ _ _ _ _] -> w363
          tunnel: [_ _ _ _ _ _ _ _ _ _ _ _ _ _ _ _ _ _ _ _ w419 _ _ _ _ _ _ _ _ _ _ _ _ _ _ _ _ _ _ _ _ _ _ _ _ _ _ _] -> w362
          tunnel: [_ _ _ _ _ _ _ _ _ _ _ _ _ _ _ _ _ _ _ _ _ w420 _ _ _ _ _ _ _ _ _ _ _ _ _ _ _ _ _ _ _ _ _ _ _ _ _ _] -> w361
          tunnel: [_ _ _ _ _ _ _ _ _ _ _ _ _ _ _ _ _ _ _ _ _ _ w421 _ _ _ _ _ _ _ _ _ _ _ _ _ _ _ _ _ _ _ _ _ _ _ _ _] -> w360
          tunnel: [_ _ _ _ _ _ _ _ _ _ _ _ _ _ _ _ _ _ _ _ _ _ _ w422 _ _ _ _ _ _ _ _ _ _ _ _ _ _ _ _ _ _ _ _ _ _ _ _] -> w359
          tunnel: [_ _ _ _ _ _ _ _ _ _ _ _ _ _ _ _ _ _ _ _ _ _ _ _ w423 _ _ _ _ _ _ _ _ _ _ _ _ _ _ _ _ _ _ _ _ _ _ _] -> w357
          tunnel: [_ _ _ _ _ _ _ _ _ _ _ _ _ _ _ _ _ _ _ _ _ _ _ _ _ w424 _ _ _ _ _ _ _ _ _ _ _ _ _ _ _ _ _ _ _ _ _ _] -> w356
          tunnel: [_ _ _ _ _ _ _ _ _ _ _ _ _ _ _ _ _ _ _ _ _ _ _ _ _ _ w425 _ _ _ _ _ _ _ _ _ _ _ _ _ _ _ _ _ _ _ _ _] -> w355
          tunnel: [_ _ _ _ _ _ _ _ _ _ _ _ _ _ _ _ _ _ _ _ _ _ _ _ _ _ _ w426 _ _ _ _ _ _ _ _ _ _ _ _ _ _ _ _ _ _ _ _] -> w354
          tunnel: [_ _ _ _ _ _ _ _ _ _ _ _ _ _ _ _ _ _ _ _ _ _ _ _ _ _ _ _ w427 _ _ _ _ _ _ _ _ _ _ _ _ _ _ _ _ _ _ _] -> w353
          tunnel: [_ _ _ _ _ _ _ _ _ _ _ _ _ _ _ _ _ _ _ _ _ _ _ _ _ _ _ _ _ w428 _ _ _ _ _ _ _ _ _ _ _ _ _ _ _ _ _ _] -> w352
          tunnel: [_ _ _ _ _ _ _ _ _ _ _ _ _ _ _ _ _ _ _ _ _ _ _ _ _ _ _ _ _ _ w429 _ _ _ _ _ _ _ _ _ _ _ _ _ _ _ _ _] -> w351
          tunnel: [_ _ _ _ _ _ _ _ _ _ _ _ _ _ _ _ _ _ _ _ _ _ _ _ _ _ _ _ _ _ _ w430 _ _ _ _ _ _ _ _ _ _ _ _ _ _ _ _] -> w350
          tunnel: [_ _ _ _ _ _ _ _ _ _ _ _ _ _ _ _ _ _ _ _ _ _ _ _ _ _ _ _ _ _ _ _ w431 _ _ _ _ _ _ _ _ _ _ _ _ _ _ _] -> w349
          tunnel: [_ _ _ _ _ _ _ _ _ _ _ _ _ _ _ _ _ _ _ _ _ _ _ _ _ _ _ _ _ _ _ _ _ w432 _ _ _ _ _ _ _ _ _ _ _ _ _ _] -> w348
          tunnel: [_ _ _ _ _ _ _ _ _ _ _ _ _ _ _ _ _ _ _ _ _ _ _ _ _ _ _ _ _ _ _ _ _ _ w433 _ _ _ _ _ _ _ _ _ _ _ _ _] -> w347
          tunnel: [_ _ _ _ _ _ _ _ _ _ _ _ _ _ _ _ _ _ _ _ _ _ _ _ _ _ _ _ _ _ _ _ _ _ _ w434 _ _ _ _ _ _ _ _ _ _ _ _] -> w346
          tunnel: [_ _ _ _ _ _ _ _ _ _ _ _ _ _ _ _ _ _ _ _ _ _ _ _ _ _ _ _ _ _ _ _ _ _ _ _ w435 _ _ _ _ _ _ _ _ _ _ _] -> w344
          tunnel: [_ _ _ _ _ _ _ _ _ _ _ _ _ _ _ _ _ _ _ _ _ _ _ _ _ _ _ _ _ _ _ _ _ _ _ _ _ w436 _ _ _ _ _ _ _ _ _ _] -> w343
          tunnel: [_ _ _ _ _ _ _ _ _ _ _ _ _ _ _ _ _ _ _ _ _ _ _ _ _ _ _ _ _ _ _ _ _ _ _ _ _ _ w437 _ _ _ _ _ _ _ _ _] -> w342
          tunnel: [_ _ _ _ _ _ _ _ _ _ _ _ _ _ _ _ _ _ _ _ _ _ _ _ _ _ _ _ _ _ _ _ _ _ _ _ _ _ _ w438 _ _ _ _ _ _ _ _] -> w341
          tunnel: [_ _ _ _ _ _ _ _ _ _ _ _ _ _ _ _ _ _ _ _ _ _ _ _ _ _ _ _ _ _ _ _ _ _ _ _ _ _ _ _ w439 _ _ _ _ _ _ _] -> w340
          tunnel: [_ _ _ _ _ _ _ _ _ _ _ _ _ _ _ _ _ _ _ _ _ _ _ _ _ _ _ _ _ _ _ _ _ _ _ _ _ _ _ _ _ w440 _ _ _ _ _ _] -> w339
          tunnel: [_ _ _ _ _ _ _ _ _ _ _ _ _ _ _ _ _ _ _ _ _ _ _ _ _ _ _ _ _ _ _ _ _ _ _ _ _ _ _ _ _ _ w441 _ _ _ _ _] -> w338
          tunnel: [_ _ _ _ _ _ _ _ _ _ _ _ _ _ _ _ _ _ _ _ _ _ _ _ _ _ _ _ _ _ _ _ _ _ _ _ _ _ _ _ _ _ _ w442 _ _ _ _] -> w337
          tunnel: [_ _ _ _ _ _ _ _ _ _ _ _ _ _ _ _ _ _ _ _ _ _ _ _ _ _ _ _ _ _ _ _ _ _ _ _ _ _ _ _ _ _ _ _ w443 _ _ _] -> w336
          tunnel: [_ _ _ _ _ _ _ _ _ _ _ _ _ _ _ _ _ _ _ _ _ _ _ _ _ _ _ _ _ _ _ _ _ _ _ _ _ _ _ _ _ _ _ _ _ w444 _ _] -> w335
          tunnel: [_ _ _ _ _ _ _ _ _ _ _ _ _ _ _ _ _ _ _ _ _ _ _ _ _ _ _ _ _ _ _ _ _ _ _ _ _ _ _ _ _ _ _ _ _ _ w445 _] -> w334
          tunnel: [_ _ _ _ _ _ _ _ _ _ _ _ _ _ _ _ _ _ _ _ _ _ _ _ _ _ _ _ _ _ _ _ _ _ _ _ _ _ _ _ _ _ _ _ _ _ _ w446] -> w333
          frame #0 {
            n363 = property on="P1 Piece" class="Pict"() -> ("Position"=w399:T1)  [unwired: 2 in, 2 out]
          }
          frame #1 {
            n364 = property on="P1 Piece 2" class="Pict"() -> ("Position"=w400:T1)  [unwired: 2 in, 2 out]
          }
          frame #2 {
            n365 = property on="P1 Piece 3" class="Pict"() -> ("Position"=w401:T1)  [unwired: 2 in, 2 out]
          }
          frame #3 {
            n366 = property on="P1 Piece 4" class="Pict"() -> ("Position"=w402:T1)  [unwired: 2 in, 2 out]
          }
          frame #4 {
            n367 = property on="P1 Piece 5" class="Pict"() -> ("Position"=w403:T1)  [unwired: 2 in, 2 out]
          }
          frame #5 {
            n368 = property on="P1 Piece 6" class="Pict"() -> ("Position"=w404:T1)  [unwired: 2 in, 2 out]
          }
          frame #6 {
            n369 = property on="P1 Piece 7" class="Pict"() -> ("Position"=w405:T1)  [unwired: 2 in, 2 out]
          }
          frame #7 {
            n370 = property on="P1 Piece 8" class="Pict"() -> ("Position"=w406:T1)  [unwired: 2 in, 2 out]
          }
          frame #8 {
            n371 = property on="P1 Piece 9" class="Pict"() -> ("Position"=w407:T1)  [unwired: 2 in, 2 out]
          }
          frame #9 {
            n372 = property on="P1 Piece 10" class="Pict"() -> ("Position"=w408:T1)  [unwired: 2 in, 2 out]
          }
          frame #10 {
            n373 = property on="P1 Piece 11" class="Pict"() -> ("Position"=w409:T1)  [unwired: 2 in, 2 out]
          }
          frame #11 {
            n374 = property on="P1 Piece 12" class="Pict"() -> ("Position"=w410:T1)  [unwired: 2 in, 2 out]
          }
          frame #12 {
            n375 = property on="P2 Piece" class="Pict"() -> ("Position"=w411:T1)  [unwired: 2 in, 2 out]
          }
          frame #13 {
            n376 = property on="P2 Piece 2" class="Pict"() -> ("Position"=w412:T1)  [unwired: 2 in, 2 out]
          }
          frame #14 {
            n377 = property on="P2 Piece 3" class="Pict"() -> ("Position"=w413:T1)  [unwired: 2 in, 2 out]
          }
          frame #15 {
            n378 = property on="P2 Piece 4" class="Pict"() -> ("Position"=w414:T1)  [unwired: 2 in, 2 out]
          }
          frame #16 {
            n379 = property on="P2 Piece 5" class="Pict"() -> ("Position"=w415:T1)  [unwired: 2 in, 2 out]
          }
          frame #17 {
            n380 = property on="P2 Piece 6" class="Pict"() -> ("Position"=w416:T1)  [unwired: 2 in, 2 out]
          }
          frame #18 {
            n381 = property on="P2 Piece 7" class="Pict"() -> ("Position"=w417:T1)  [unwired: 2 in, 2 out]
          }
          frame #19 {
            n382 = property on="P2 Piece 8" class="Pict"() -> ("Position"=w418:T1)  [unwired: 2 in, 2 out]
          }
          frame #20 {
            n383 = property on="P2 Piece 9" class="Pict"() -> ("Position"=w419:T1)  [unwired: 2 in, 2 out]
          }
          frame #21 {
            n384 = property on="P2 Piece 10" class="Pict"() -> ("Position"=w420:T1)  [unwired: 2 in, 2 out]
          }
          frame #22 {
            n385 = property on="P2 Piece 11" class="Pict"() -> ("Position"=w421:T1)  [unwired: 2 in, 2 out]
          }
          frame #23 {
            n386 = property on="P2 Piece 12" class="Pict"() -> ("Position"=w422:T1)  [unwired: 2 in, 2 out]
          }
          frame #24 {
            n387 = property on="P1 King" class="Pict"() -> ("Position"=w423:T1)  [unwired: 2 in, 2 out]
          }
          frame #25 {
            n388 = property on="P1 King 2" class="Pict"() -> ("Position"=w424:T1)  [unwired: 2 in, 2 out]
          }
          frame #26 {
            n389 = property on="P1 King 3" class="Pict"() -> ("Position"=w425:T1)  [unwired: 2 in, 2 out]
          }
          frame #27 {
            n390 = property on="P1 King 4" class="Pict"() -> ("Position"=w426:T1)  [unwired: 2 in, 2 out]
          }
          frame #28 {
            n391 = property on="P1 King 5" class="Pict"() -> ("Position"=w427:T1)  [unwired: 2 in, 2 out]
          }
          frame #29 {
            n392 = property on="P1 King 6" class="Pict"() -> ("Position"=w428:T1)  [unwired: 2 in, 2 out]
          }
          frame #30 {
            n393 = property on="P1 King 7" class="Pict"() -> ("Position"=w429:T1)  [unwired: 2 in, 2 out]
          }
          frame #31 {
            n394 = property on="P1 King 8" class="Pict"() -> ("Position"=w430:T1)  [unwired: 2 in, 2 out]
          }
          frame #32 {
            n395 = property on="P1 King 9" class="Pict"() -> ("Position"=w431:T1)  [unwired: 2 in, 2 out]
          }
          frame #33 {
            n396 = property on="P1 King 10" class="Pict"() -> ("Position"=w432:T1)  [unwired: 2 in, 2 out]
          }
          frame #34 {
            n397 = property on="P1 King 11" class="Pict"() -> ("Position"=w433:T1)  [unwired: 2 in, 2 out]
          }
          frame #35 {
            n398 = property on="P1 King 12" class="Pict"() -> ("Position"=w434:T1)  [unwired: 2 in, 2 out]
          }
          frame #36 {
            n399 = property on="P2 King" class="Pict"() -> ("Position"=w435:T1)  [unwired: 2 in, 2 out]
          }
          frame #37 {
            n400 = property on="P2 King 2" class="Pict"() -> ("Position"=w436:T1)  [unwired: 2 in, 2 out]
          }
          frame #38 {
            n401 = property on="P2 King 3" class="Pict"() -> ("Position"=w437:T1)  [unwired: 2 in, 2 out]
          }
          frame #39 {
            n402 = property on="P2 King 4" class="Pict"() -> ("Position"=w438:T1)  [unwired: 2 in, 2 out]
          }
          frame #40 {
            n403 = property on="P2 King 5" class="Pict"() -> ("Position"=w439:T1)  [unwired: 2 in, 2 out]
          }
          frame #41 {
            n404 = property on="P2 King 6" class="Pict"() -> ("Position"=w440:T1)  [unwired: 2 in, 2 out]
          }
          frame #42 {
            n405 = property on="P2 King 7" class="Pict"() -> ("Position"=w441:T1)  [unwired: 2 in, 2 out]
          }
          frame #43 {
            n406 = property on="P2 King 8" class="Pict"() -> ("Position"=w442:T1)  [unwired: 2 in, 2 out]
          }
          frame #44 {
            n407 = property on="P2 King 9" class="Pict"() -> ("Position"=w443:T1)  [unwired: 2 in, 2 out]
          }
          frame #45 {
            n408 = property on="P2 King 10" class="Pict"() -> ("Position"=w444:T1)  [unwired: 2 in, 2 out]
          }
          frame #46 {
            n409 = property on="P2 King 11" class="Pict"() -> ("Position"=w445:T1)  [unwired: 2 in, 2 out]
          }
          frame #47 {
            n410 = property on="P2 King 12" class="Pict"() -> ("Position"=w446:T1)  [unwired: 2 in, 2 out]
          }
        }
        n411 = Build Array(w383, w382, w381, w380, w379, w378, w377, w376, w375, w374, w373, w372) -> (w371:T1[])
        n412 = Build Array (concatenate)(w371, w370, w369, w368, w367, w366, w365, w364, w363, w362, w361, w360, w359) -> (w358:T1[])
        n413 = Build Array (concatenate)(w358, w357, w356, w355, w354, w353, w352, w351, w350, w349, w348, w347, w346) -> (w345:T1[])
        n414 = Build Array (concatenate)(w345, w344, w343, w342, w341, w340, w339, w338, w337, w336, w335, w334, w333) -> (w332:T1[])
        n415 = for {
          tunnel: w332 -> [w454] mode=indexing
          tunnel: w396 -> [w453]
          n416 = Unbundle(w454) -> ("Left"=w448:i32, "Top"=w447:i32)
          n417 = Set File Position(refnum=w453, from (0:start)=enum16{"start", "end", "current"}."end") -> (refnum out=w450:refnum<file>)  [unwired: 2 in, 1 out]
          n418 = Format Into String(initial string=w450, " " ("input 1")) -> (resulting string=w449:refnum<file>)  [unwired: 2 in, 1 out]
          n419 = Format Into String(initial string=w449, w448, w447) -> ()  [unwired: 2 in, 2 out]
        }
      }
      event "Save and Quit": Value Change {
        n420 = event-data() -> ()  [unwired: 1 in, 6 out]
        n421 = flat-sequence {
          tunnel: [w455] -> _
          frame #0 {
            n422 = global read "Game Info Global Variable.vi" "P1 King Text Green Color"() -> (w464:i32)
            n423 = global read "Game Info Global Variable.vi" "P2 King Text Green Color"() -> (w458:i32)
            n424 = global read "Game Info Global Variable.vi" "P1 King Text Blue Color"() -> (w463:i32)
            n425 = global read "Game Info Global Variable.vi" "P2 King Text Blue Color"() -> (w457:i32)
            n426 = global read "Game Info Global Variable.vi" "P1 King Text Red Color"() -> (w465:i32)
            n427 = global read "Game Info Global Variable.vi" "P2 King Text Red Color"() -> (w459:i32)
            n428 = global read "Game Info Global Variable.vi" "P1 Green Color"() -> (w467:i32)
            n429 = global read "Game Info Global Variable.vi" "P2 Green Color"() -> (w461:i32)
            n430 = local read "Player 1 Name"() -> (w470:string)
            n431 = local read "Player 2 Name"() -> (w469:string)
            n432 = global read "Game Info Global Variable.vi" "P1 Red Color"() -> (w468:i32)
            n433 = global read "Game Info Global Variable.vi" "P1 Blue Color"() -> (w466:i32)
            n434 = global read "Game Info Global Variable.vi" "P2 Blue Color"() -> (w460:i32)
            n435 = global read "Game Info Global Variable.vi" "P2 Red Color"() -> (w462:i32)
            n436 = Format Into String(w470, w469, w468, w467, w466, w465, w464, w463, w462, w461, w460, w459, w458, w457) -> (resulting string=w456:refnum<file>)  [unwired: 3 in, 1 out]
            n437 = stacked-sequence {
              tunnel: [w522 _ _ _ _ _ _ _ _ _ _ _ _ _ _ _ _ _ _ _ _ _ _ _ _ _ _ _ _ _ _ _ _ _ _ _ _ _ _ _ _ _ _ _ _ _ _ _] -> w471
              tunnel: [_ w523 _ _ _ _ _ _ _ _ _ _ _ _ _ _ _ _ _ _ _ _ _ _ _ _ _ _ _ _ _ _ _ _ _ _ _ _ _ _ _ _ _ _ _ _ _ _] -> w472
              tunnel: [_ _ w524 _ _ _ _ _ _ _ _ _ _ _ _ _ _ _ _ _ _ _ _ _ _ _ _ _ _ _ _ _ _ _ _ _ _ _ _ _ _ _ _ _ _ _ _ _] -> w473
              tunnel: [_ _ _ w525 _ _ _ _ _ _ _ _ _ _ _ _ _ _ _ _ _ _ _ _ _ _ _ _ _ _ _ _ _ _ _ _ _ _ _ _ _ _ _ _ _ _ _ _] -> w474
              tunnel: [_ _ _ _ w526 _ _ _ _ _ _ _ _ _ _ _ _ _ _ _ _ _ _ _ _ _ _ _ _ _ _ _ _ _ _ _ _ _ _ _ _ _ _ _ _ _ _ _] -> w475
              tunnel: [_ _ _ _ _ w527 _ _ _ _ _ _ _ _ _ _ _ _ _ _ _ _ _ _ _ _ _ _ _ _ _ _ _ _ _ _ _ _ _ _ _ _ _ _ _ _ _ _] -> w476
              tunnel: [_ _ _ _ _ _ w528 _ _ _ _ _ _ _ _ _ _ _ _ _ _ _ _ _ _ _ _ _ _ _ _ _ _ _ _ _ _ _ _ _ _ _ _ _ _ _ _ _] -> w477
              tunnel: [_ _ _ _ _ _ _ w529 _ _ _ _ _ _ _ _ _ _ _ _ _ _ _ _ _ _ _ _ _ _ _ _ _ _ _ _ _ _ _ _ _ _ _ _ _ _ _ _] -> w478
              tunnel: [_ _ _ _ _ _ _ _ w530 _ _ _ _ _ _ _ _ _ _ _ _ _ _ _ _ _ _ _ _ _ _ _ _ _ _ _ _ _ _ _ _ _ _ _ _ _ _ _] -> w479
              tunnel: [_ _ _ _ _ _ _ _ _ w531 _ _ _ _ _ _ _ _ _ _ _ _ _ _ _ _ _ _ _ _ _ _ _ _ _ _ _ _ _ _ _ _ _ _ _ _ _ _] -> w480
              tunnel: [_ _ _ _ _ _ _ _ _ _ w532 _ _ _ _ _ _ _ _ _ _ _ _ _ _ _ _ _ _ _ _ _ _ _ _ _ _ _ _ _ _ _ _ _ _ _ _ _] -> w481
              tunnel: [_ _ _ _ _ _ _ _ _ _ _ w533 _ _ _ _ _ _ _ _ _ _ _ _ _ _ _ _ _ _ _ _ _ _ _ _ _ _ _ _ _ _ _ _ _ _ _ _] -> w482
              tunnel: [_ _ _ _ _ _ _ _ _ _ _ _ w534 _ _ _ _ _ _ _ _ _ _ _ _ _ _ _ _ _ _ _ _ _ _ _ _ _ _ _ _ _ _ _ _ _ _ _] -> w484
              tunnel: [_ _ _ _ _ _ _ _ _ _ _ _ _ w535 _ _ _ _ _ _ _ _ _ _ _ _ _ _ _ _ _ _ _ _ _ _ _ _ _ _ _ _ _ _ _ _ _ _] -> w485
              tunnel: [_ _ _ _ _ _ _ _ _ _ _ _ _ _ w536 _ _ _ _ _ _ _ _ _ _ _ _ _ _ _ _ _ _ _ _ _ _ _ _ _ _ _ _ _ _ _ _ _] -> w486
              tunnel: [_ _ _ _ _ _ _ _ _ _ _ _ _ _ _ w537 _ _ _ _ _ _ _ _ _ _ _ _ _ _ _ _ _ _ _ _ _ _ _ _ _ _ _ _ _ _ _ _] -> w487
              tunnel: [_ _ _ _ _ _ _ _ _ _ _ _ _ _ _ _ w538 _ _ _ _ _ _ _ _ _ _ _ _ _ _ _ _ _ _ _ _ _ _ _ _ _ _ _ _ _ _ _] -> w488
              tunnel: [_ _ _ _ _ _ _ _ _ _ _ _ _ _ _ _ _ w539 _ _ _ _ _ _ _ _ _ _ _ _ _ _ _ _ _ _ _ _ _ _ _ _ _ _ _ _ _ _] -> w489
              tunnel: [_ _ _ _ _ _ _ _ _ _ _ _ _ _ _ _ _ _ w540 _ _ _ _ _ _ _ _ _ _ _ _ _ _ _ _ _ _ _ _ _ _ _ _ _ _ _ _ _] -> w490
              tunnel: [_ _ _ _ _ _ _ _ _ _ _ _ _ _ _ _ _ _ _ w541 _ _ _ _ _ _ _ _ _ _ _ _ _ _ _ _ _ _ _ _ _ _ _ _ _ _ _ _] -> w491
              tunnel: [_ _ _ _ _ _ _ _ _ _ _ _ _ _ _ _ _ _ _ _ w542 _ _ _ _ _ _ _ _ _ _ _ _ _ _ _ _ _ _ _ _ _ _ _ _ _ _ _] -> w492
              tunnel: [_ _ _ _ _ _ _ _ _ _ _ _ _ _ _ _ _ _ _ _ _ w543 _ _ _ _ _ _ _ _ _ _ _ _ _ _ _ _ _ _ _ _ _ _ _ _ _ _] -> w493
              tunnel: [_ _ _ _ _ _ _ _ _ _ _ _ _ _ _ _ _ _ _ _ _ _ w544 _ _ _ _ _ _ _ _ _ _ _ _ _ _ _ _ _ _ _ _ _ _ _ _ _] -> w495
              tunnel: [_ _ _ _ _ _ _ _ _ _ _ _ _ _ _ _ _ _ _ _ _ _ _ w545 _ _ _ _ _ _ _ _ _ _ _ _ _ _ _ _ _ _ _ _ _ _ _ _] -> w494
              tunnel: [_ _ _ _ _ _ _ _ _ _ _ _ _ _ _ _ _ _ _ _ _ _ _ _ w546 _ _ _ _ _ _ _ _ _ _ _ _ _ _ _ _ _ _ _ _ _ _ _] -> w498
              tunnel: [_ _ _ _ _ _ _ _ _ _ _ _ _ _ _ _ _ _ _ _ _ _ _ _ _ w547 _ _ _ _ _ _ _ _ _ _ _ _ _ _ _ _ _ _ _ _ _ _] -> w499
              tunnel: [_ _ _ _ _ _ _ _ _ _ _ _ _ _ _ _ _ _ _ _ _ _ _ _ _ _ w548 _ _ _ _ _ _ _ _ _ _ _ _ _ _ _ _ _ _ _ _ _] -> w500
              tunnel: [_ _ _ _ _ _ _ _ _ _ _ _ _ _ _ _ _ _ _ _ _ _ _ _ _ _ _ w549 _ _ _ _ _ _ _ _ _ _ _ _ _ _ _ _ _ _ _ _] -> w501
              tunnel: [_ _ _ _ _ _ _ _ _ _ _ _ _ _ _ _ _ _ _ _ _ _ _ _ _ _ _ _ w550 _ _ _ _ _ _ _ _ _ _ _ _ _ _ _ _ _ _ _] -> w502
              tunnel: [_ _ _ _ _ _ _ _ _ _ _ _ _ _ _ _ _ _ _ _ _ _ _ _ _ _ _ _ _ w551 _ _ _ _ _ _ _ _ _ _ _ _ _ _ _ _ _ _] -> w503
              tunnel: [_ _ _ _ _ _ _ _ _ _ _ _ _ _ _ _ _ _ _ _ _ _ _ _ _ _ _ _ _ _ w552 _ _ _ _ _ _ _ _ _ _ _ _ _ _ _ _ _] -> w504
              tunnel: [_ _ _ _ _ _ _ _ _ _ _ _ _ _ _ _ _ _ _ _ _ _ _ _ _ _ _ _ _ _ _ w553 _ _ _ _ _ _ _ _ _ _ _ _ _ _ _ _] -> w505
              tunnel: [_ _ _ _ _ _ _ _ _ _ _ _ _ _ _ _ _ _ _ _ _ _ _ _ _ _ _ _ _ _ _ _ w554 _ _ _ _ _ _ _ _ _ _ _ _ _ _ _] -> w506
              tunnel: [_ _ _ _ _ _ _ _ _ _ _ _ _ _ _ _ _ _ _ _ _ _ _ _ _ _ _ _ _ _ _ _ _ w555 _ _ _ _ _ _ _ _ _ _ _ _ _ _] -> w507
              tunnel: [_ _ _ _ _ _ _ _ _ _ _ _ _ _ _ _ _ _ _ _ _ _ _ _ _ _ _ _ _ _ _ _ _ _ w556 _ _ _ _ _ _ _ _ _ _ _ _ _] -> w508
              tunnel: [_ _ _ _ _ _ _ _ _ _ _ _ _ _ _ _ _ _ _ _ _ _ _ _ _ _ _ _ _ _ _ _ _ _ _ w557 _ _ _ _ _ _ _ _ _ _ _ _] -> w509
              tunnel: [_ _ _ _ _ _ _ _ _ _ _ _ _ _ _ _ _ _ _ _ _ _ _ _ _ _ _ _ _ _ _ _ _ _ _ _ w558 _ _ _ _ _ _ _ _ _ _ _] -> w510
              tunnel: [_ _ _ _ _ _ _ _ _ _ _ _ _ _ _ _ _ _ _ _ _ _ _ _ _ _ _ _ _ _ _ _ _ _ _ _ _ w559 _ _ _ _ _ _ _ _ _ _] -> w511
              tunnel: [_ _ _ _ _ _ _ _ _ _ _ _ _ _ _ _ _ _ _ _ _ _ _ _ _ _ _ _ _ _ _ _ _ _ _ _ _ _ w560 _ _ _ _ _ _ _ _ _] -> w512
              tunnel: [_ _ _ _ _ _ _ _ _ _ _ _ _ _ _ _ _ _ _ _ _ _ _ _ _ _ _ _ _ _ _ _ _ _ _ _ _ _ _ w561 _ _ _ _ _ _ _ _] -> w513
              tunnel: [_ _ _ _ _ _ _ _ _ _ _ _ _ _ _ _ _ _ _ _ _ _ _ _ _ _ _ _ _ _ _ _ _ _ _ _ _ _ _ _ w562 _ _ _ _ _ _ _] -> w514
              tunnel: [_ _ _ _ _ _ _ _ _ _ _ _ _ _ _ _ _ _ _ _ _ _ _ _ _ _ _ _ _ _ _ _ _ _ _ _ _ _ _ _ _ w563 _ _ _ _ _ _] -> w515
              tunnel: [_ _ _ _ _ _ _ _ _ _ _ _ _ _ _ _ _ _ _ _ _ _ _ _ _ _ _ _ _ _ _ _ _ _ _ _ _ _ _ _ _ _ w564 _ _ _ _ _] -> w516
              tunnel: [_ _ _ _ _ _ _ _ _ _ _ _ _ _ _ _ _ _ _ _ _ _ _ _ _ _ _ _ _ _ _ _ _ _ _ _ _ _ _ _ _ _ _ w565 _ _ _ _] -> w517
              tunnel: [_ _ _ _ _ _ _ _ _ _ _ _ _ _ _ _ _ _ _ _ _ _ _ _ _ _ _ _ _ _ _ _ _ _ _ _ _ _ _ _ _ _ _ _ w566 _ _ _] -> w518
              tunnel: [_ _ _ _ _ _ _ _ _ _ _ _ _ _ _ _ _ _ _ _ _ _ _ _ _ _ _ _ _ _ _ _ _ _ _ _ _ _ _ _ _ _ _ _ _ w567 _ _] -> w519
              tunnel: [_ _ _ _ _ _ _ _ _ _ _ _ _ _ _ _ _ _ _ _ _ _ _ _ _ _ _ _ _ _ _ _ _ _ _ _ _ _ _ _ _ _ _ _ _ _ w568 _] -> w520
              tunnel: [_ _ _ _ _ _ _ _ _ _ _ _ _ _ _ _ _ _ _ _ _ _ _ _ _ _ _ _ _ _ _ _ _ _ _ _ _ _ _ _ _ _ _ _ _ _ _ w569] -> w521
              frame #0 {
                n438 = property on="P1 Piece" class="Pict"() -> ("Position"=w522:T1)  [unwired: 2 in, 2 out]
              }
              frame #1 {
                n439 = property on="P1 Piece 2" class="Pict"() -> ("Position"=w523:T1)  [unwired: 2 in, 2 out]
              }
              frame #2 {
                n440 = property on="P1 Piece 3" class="Pict"() -> ("Position"=w524:T1)  [unwired: 2 in, 2 out]
              }
              frame #3 {
                n441 = property on="P1 Piece 4" class="Pict"() -> ("Position"=w525:T1)  [unwired: 2 in, 2 out]
              }
              frame #4 {
                n442 = property on="P1 Piece 5" class="Pict"() -> ("Position"=w526:T1)  [unwired: 2 in, 2 out]
              }
              frame #5 {
                n443 = property on="P1 Piece 6" class="Pict"() -> ("Position"=w527:T1)  [unwired: 2 in, 2 out]
              }
              frame #6 {
                n444 = property on="P1 Piece 7" class="Pict"() -> ("Position"=w528:T1)  [unwired: 2 in, 2 out]
              }
              frame #7 {
                n445 = property on="P1 Piece 8" class="Pict"() -> ("Position"=w529:T1)  [unwired: 2 in, 2 out]
              }
              frame #8 {
                n446 = property on="P1 Piece 9" class="Pict"() -> ("Position"=w530:T1)  [unwired: 2 in, 2 out]
              }
              frame #9 {
                n447 = property on="P1 Piece 10" class="Pict"() -> ("Position"=w531:T1)  [unwired: 2 in, 2 out]
              }
              frame #10 {
                n448 = property on="P1 Piece 11" class="Pict"() -> ("Position"=w532:T1)  [unwired: 2 in, 2 out]
              }
              frame #11 {
                n449 = property on="P1 Piece 12" class="Pict"() -> ("Position"=w533:T1)  [unwired: 2 in, 2 out]
              }
              frame #12 {
                n450 = property on="P2 Piece" class="Pict"() -> ("Position"=w534:T1)  [unwired: 2 in, 2 out]
              }
              frame #13 {
                n451 = property on="P2 Piece 2" class="Pict"() -> ("Position"=w535:T1)  [unwired: 2 in, 2 out]
              }
              frame #14 {
                n452 = property on="P2 Piece 3" class="Pict"() -> ("Position"=w536:T1)  [unwired: 2 in, 2 out]
              }
              frame #15 {
                n453 = property on="P2 Piece 4" class="Pict"() -> ("Position"=w537:T1)  [unwired: 2 in, 2 out]
              }
              frame #16 {
                n454 = property on="P2 Piece 5" class="Pict"() -> ("Position"=w538:T1)  [unwired: 2 in, 2 out]
              }
              frame #17 {
                n455 = property on="P2 Piece 6" class="Pict"() -> ("Position"=w539:T1)  [unwired: 2 in, 2 out]
              }
              frame #18 {
                n456 = property on="P2 Piece 7" class="Pict"() -> ("Position"=w540:T1)  [unwired: 2 in, 2 out]
              }
              frame #19 {
                n457 = property on="P2 Piece 8" class="Pict"() -> ("Position"=w541:T1)  [unwired: 2 in, 2 out]
              }
              frame #20 {
                n458 = property on="P2 Piece 9" class="Pict"() -> ("Position"=w542:T1)  [unwired: 2 in, 2 out]
              }
              frame #21 {
                n459 = property on="P2 Piece 10" class="Pict"() -> ("Position"=w543:T1)  [unwired: 2 in, 2 out]
              }
              frame #22 {
                n460 = property on="P2 Piece 11" class="Pict"() -> ("Position"=w544:T1)  [unwired: 2 in, 2 out]
              }
              frame #23 {
                n461 = property on="P2 Piece 12" class="Pict"() -> ("Position"=w545:T1)  [unwired: 2 in, 2 out]
              }
              frame #24 {
                n462 = property on="P1 King" class="Pict"() -> ("Position"=w546:T1)  [unwired: 2 in, 2 out]
              }
              frame #25 {
                n463 = property on="P1 King 2" class="Pict"() -> ("Position"=w547:T1)  [unwired: 2 in, 2 out]
              }
              frame #26 {
                n464 = property on="P1 King 3" class="Pict"() -> ("Position"=w548:T1)  [unwired: 2 in, 2 out]
              }
              frame #27 {
                n465 = property on="P1 King 4" class="Pict"() -> ("Position"=w549:T1)  [unwired: 2 in, 2 out]
              }
              frame #28 {
                n466 = property on="P1 King 5" class="Pict"() -> ("Position"=w550:T1)  [unwired: 2 in, 2 out]
              }
              frame #29 {
                n467 = property on="P1 King 6" class="Pict"() -> ("Position"=w551:T1)  [unwired: 2 in, 2 out]
              }
              frame #30 {
                n468 = property on="P1 King 7" class="Pict"() -> ("Position"=w552:T1)  [unwired: 2 in, 2 out]
              }
              frame #31 {
                n469 = property on="P1 King 8" class="Pict"() -> ("Position"=w553:T1)  [unwired: 2 in, 2 out]
              }
              frame #32 {
                n470 = property on="P1 King 9" class="Pict"() -> ("Position"=w554:T1)  [unwired: 2 in, 2 out]
              }
              frame #33 {
                n471 = property on="P1 King 10" class="Pict"() -> ("Position"=w555:T1)  [unwired: 2 in, 2 out]
              }
              frame #34 {
                n472 = property on="P1 King 11" class="Pict"() -> ("Position"=w556:T1)  [unwired: 2 in, 2 out]
              }
              frame #35 {
                n473 = property on="P1 King 12" class="Pict"() -> ("Position"=w557:T1)  [unwired: 2 in, 2 out]
              }
              frame #36 {
                n474 = property on="P2 King" class="Pict"() -> ("Position"=w558:T1)  [unwired: 2 in, 2 out]
              }
              frame #37 {
                n475 = property on="P2 King 2" class="Pict"() -> ("Position"=w559:T1)  [unwired: 2 in, 2 out]
              }
              frame #38 {
                n476 = property on="P2 King 3" class="Pict"() -> ("Position"=w560:T1)  [unwired: 2 in, 2 out]
              }
              frame #39 {
                n477 = property on="P2 King 4" class="Pict"() -> ("Position"=w561:T1)  [unwired: 2 in, 2 out]
              }
              frame #40 {
                n478 = property on="P2 King 5" class="Pict"() -> ("Position"=w562:T1)  [unwired: 2 in, 2 out]
              }
              frame #41 {
                n479 = property on="P2 King 6" class="Pict"() -> ("Position"=w563:T1)  [unwired: 2 in, 2 out]
              }
              frame #42 {
                n480 = property on="P2 King 7" class="Pict"() -> ("Position"=w564:T1)  [unwired: 2 in, 2 out]
              }
              frame #43 {
                n481 = property on="P2 King 8" class="Pict"() -> ("Position"=w565:T1)  [unwired: 2 in, 2 out]
              }
              frame #44 {
                n482 = property on="P2 King 9" class="Pict"() -> ("Position"=w566:T1)  [unwired: 2 in, 2 out]
              }
              frame #45 {
                n483 = property on="P2 King 10" class="Pict"() -> ("Position"=w567:T1)  [unwired: 2 in, 2 out]
              }
              frame #46 {
                n484 = property on="P2 King 11" class="Pict"() -> ("Position"=w568:T1)  [unwired: 2 in, 2 out]
              }
              frame #47 {
                n485 = property on="P2 King 12" class="Pict"() -> ("Position"=w569:T1)  [unwired: 2 in, 2 out]
              }
            }
            n486 = Build Array(w471, w472, w473, w474, w475, w476, w477, w478, w479, w480, w481, w482) -> (w483:T1[])
            n487 = Build Array (concatenate)(w483, w484, w485, w486, w487, w488, w489, w490, w491, w492, w493, w495, w494) -> (w496:T1[])
            n488 = Build Array (concatenate)(w496, w498, w499, w500, w501, w502, w503, w504, w505, w506, w507, w508, w509) -> (w497:T1[])
            n489 = Build Array (concatenate)(w497, w510, w511, w512, w513, w514, w515, w516, w517, w518, w519, w520, w521) -> (w455:T1[])
            n490 = for {
              tunnel: w455 -> [w577] mode=indexing
              tunnel: w456 -> [w576]
              n491 = Unbundle(w577) -> ("Left"=w571:i32, "Top"=w570:i32)
              n492 = Set File Position(refnum=w576, from (0:start)=enum16{"start", "end", "current"}."end") -> (refnum out=w573:refnum<file>)  [unwired: 2 in, 1 out]
              n493 = Format Into String(initial string=w573, " " ("input 1")) -> (resulting string=w572:refnum<file>)  [unwired: 2 in, 1 out]
              n494 = Format Into String(initial string=w572, w571, w570) -> ()  [unwired: 2 in, 2 out]
            }
          }
          frame #1 {
            n495 = vi-ref "Checkers Main Menu.vi"() -> (w581:refnum<vi>)
            n496 = vi-ref "Checkers Gymnopedie Music Player.vi"() -> (w578:refnum<vi>)
            n497 = invoke class="VI" method="Run VI"(reference=w581, "Wait until done"=FALSE ("Wait Until Done")) -> (reference out=w582:refnum<vi>, error out=w583:errorcluster)  [unwired: 3 in, 3 out]
            n498 = invoke class="VI" method="Run VI"(reference=w578, "Wait until done"=FALSE ("Wait Until Done")) -> ()  [unwired: 3 in, 5 out]
            n499 = invoke class="VI" method="FP.Open"(reference=w582, error in=w583, "Activate"=TRUE ("Activate?")) -> (error out=w584:errorcluster)  [unwired: 2 in, 4 out]
            n500 = vi-ref "Checkers Palladio Music Player.vi"() -> (w580:refnum<vi>)
            n501 = vi-ref "Checkers PvP.vi"() -> (w585:refnum<vi>)
            n502 = invoke class="VI" method="Abort VI"(reference=w585, error in=w584) -> ()  [unwired: 1 in, 3 out]
            n503 = invoke class="VI" method="Abort VI"(reference=w580) -> ()  [unwired: 2 in, 3 out]
          }
        }
      }
      event "Quit": Value Change {
        n504 = event-data() -> ()  [unwired: 1 in, 6 out]
        n505 = Two Button Dialog(message="Are you sure you want to quit without saving?", 1:"No" ("F button name (\"Cancel\")"), 2:"Yes" ("T button name (\"OK\")")) -> (T button?=w588:bool)
        n506 = case shown="False" w588 {
          frame False {
            # "Player changed mind to quit without saving. Do nothing."
          }
          frame True {
            n507 = vi-ref "Checkers Gymnopedie Music Player.vi"() -> (w592:refnum<vi>)
            n508 = vi-ref "Checkers Main Menu.vi"() -> (w601:refnum<vi>)
            n509 = invoke class="VI" method="Run VI"(reference=w601, "Wait until done"=FALSE ("Wait Until Done")) -> (reference out=w600:refnum<vi>, error out=w599:errorcluster)  [unwired: 3 in, 3 out]
            n510 = invoke class="VI" method="Run VI"(reference=w592, "Wait until done"=FALSE ("Wait Until Done")) -> ()  [unwired: 3 in, 5 out]
            n511 = invoke class="VI" method="FP.Open"(reference=w600, error in=w599, "Activate"=TRUE ("Activate?")) -> (error out=w598:errorcluster)  [unwired: 2 in, 4 out]
            n512 = vi-ref "Checkers Palladio Music Player.vi"() -> (w594:refnum<vi>)
            n513 = vi-ref "Checkers PvP.vi"() -> (w597:refnum<vi>)
            n514 = invoke class="VI" method="Abort VI"(reference=w597, error in=w598) -> ()  [unwired: 1 in, 3 out]
            n515 = invoke class="VI" method="Abort VI"(reference=w594) -> ()  [unwired: 2 in, 3 out]
          }
        }
      }
      event "P1 Piece", "P1 Piece 2", "P1 Piece 3", "P1 Piece 4", "P1 Piece 5", "P1 Piece 6", "P1 Piece 7", "P1 Piece 8", "P1 Piece 9", "P1 Piece 10", "P1 Piece 11", "P1 Piece 12": Mouse Down {
        n516 = event-data() -> ("CtlRef"=w605:refnum<vi>)  [unwired: 1 in, 7 out]
        n517 = local read "P1 Turn Light"() -> (w606:bool)
        n518 = case shown="True" w606 {
          tunnel: w605 -> [_ w612]
          tunnel: [_ w607] -> w604
          tunnel: [_ w610] -> w603
          tunnel: [_ w608] -> w602
          frame False {
            # "It's not player 1's turn yet. Do nothing."
          }
          frame True {
            # "At this point, I use an \nequation to turn the pixel\ncoordinates into the array coordinates\nof the piece that the user clicked."
            # "Left first"
            # "row[0], collumn[1]"
            n519 = property on="Property Node" class="Pict"(reference=w612) -> ("Position"=w608:T1)  [unwired: 1 in, 2 out]
            n520 = global read "Board Layout Global Variable.vi" "Board Layout"() -> (w639:dbl[][])
            n521 = Unbundle By Name(w608) -> ("Left"=w629:i32, "Top"=w627:i32)
            n522 = expression code="(x-469)/42"(w629) -> (w630:i32)
            n523 = expression code="(x-56)/42"(w627) -> (w628:i32)
            n524 = To Long Integer(number=w630) -> (32bit integer=w613:i32)
            n525 = To Long Integer(number=w628) -> (32bit integer=w614:i32)
            n526 = Build Array(w614, w613) -> (w638:i32[])
            n527 = call "MoveLogic.vi"("Coordinates"=w638, "Array"=w639) -> ("Moves"=w635:dbl[][])
            n528 = Index Array(array=w635, index (row)=0) -> (element=w607:dbl[])  [unwired: 1 in]
            n529 = Index Array(array=w635, index (row)=1) -> (element=w610:dbl[])  [unwired: 1 in]
            n530 = Index Array(array=w610, index=1) -> (element=w626:dbl)
            n531 = Index Array(array=w610, index=0) -> (element=w625:dbl)
            n532 = Index Array(array=w607, index=0) -> (element=w615:dbl)
            n533 = Index Array(array=w607, index=1) -> (element=w616:dbl)
            n534 = expression code="(x*42)+56"(w625) -> (w624:dbl)
            n535 = expression code="(x*42)+469"(w626) -> (w623:dbl)
            n536 = expression code="(x*42)+56"(w615) -> (w617:dbl)
            n537 = expression code="(x*42)+469"(w616) -> (w618:dbl)
            n538 = To Long Integer(number=w623) -> (32bit integer=w622:i32)
            n539 = To Long Integer(number=w624) -> (32bit integer=w621:i32)
            n540 = To Long Integer(number=w618) -> (32bit integer=w619:i32)
            n541 = To Long Integer(number=w617) -> (32bit integer=w620:i32)
            n542 = Bundle(w622, w621) -> (w609:cluster{i32, i32})  [unwired: 1 in]
            n543 = Bundle(w619, w620) -> (w611:cluster{i32, i32})  [unwired: 1 in]
            n544 = property on="P1 Top Right Marker" class="Pict"("Position"=w609) -> ()  [unwired: 2 in, 2 out]
            n545 = property on="P1 Top Left Marker" class="Pict"("Position"=w611) -> ()  [unwired: 2 in, 2 out]
          }
        }
      }
      event "P1 King", "P1 King 2", "P1 King 3", "P1 King 4", "P1 King 5", "P1 King 6", "P1 King 7", "P1 King 8", "P1 King 9", "P1 King 10", "P1 King 11", "P1 King 12": Mouse Down {
        n546 = event-data() -> ("CtlRef"=w640:refnum<vi>)  [unwired: 1 in, 7 out]
        n547 = local read "P1 Turn Light"() -> (w641:bool)
        n548 = case shown="True" w641 {
          tunnel: w640 -> [_ w642]
          frame False {
            # "It's not player 1's turn yet. Do nothing."
          }
          frame True {
            # "At this point, I use an \nequation to turn the pixel\ncoordinates into the array coordinates\nof the piece that the user clicked."
            # "Left first"
            # "row[0], collumn[1]"
            n549 = property on="Property Node" class="Pict"(reference=w642) -> ("Position"=w643:T1)  [unwired: 1 in, 2 out]
            n550 = global read "Board Layout Global Variable.vi" "Board Layout"() -> (w674:dbl[][])
            n551 = Unbundle By Name(w643) -> ("Left"=w663:i32, "Top"=w661:i32)
            n552 = expression code="(x-469)/42"(w663) -> (w664:i32)
            n553 = expression code="(x-56)/42"(w661) -> (w662:i32)
            n554 = To Long Integer(number=w664) -> (32bit integer=w646:i32)
            n555 = To Long Integer(number=w662) -> (32bit integer=w647:i32)
            n556 = Build Array(w647, w646) -> (w673:i32[])
            n557 = call "MoveLogic.vi"("Coordinates"=w673, "Array"=w674) -> ("Moves"=w670:dbl[][])
            n558 = Index Array(array=w670, index (row)=0) -> (element=w648:dbl[])  [unwired: 1 in]
            n559 = Index Array(array=w670, index (row)=1) -> (element=w667:dbl[])  [unwired: 1 in]
            n560 = Index Array(array=w667, index=1) -> (element=w660:dbl)
            n561 = Index Array(array=w667, index=0) -> (element=w659:dbl)
            n562 = Index Array(array=w648, index=0) -> (element=w649:dbl)
            n563 = Index Array(array=w648, index=1) -> (element=w650:dbl)
            n564 = expression code="(x*42)+56"(w659) -> (w658:dbl)
            n565 = expression code="(x*42)+469"(w660) -> (w657:dbl)
            n566 = expression code="(x*42)+56"(w649) -> (w651:dbl)
            n567 = expression code="(x*42)+469"(w650) -> (w652:dbl)
            n568 = To Long Integer(number=w657) -> (32bit integer=w656:i32)
            n569 = To Long Integer(number=w658) -> (32bit integer=w655:i32)
            n570 = To Long Integer(number=w652) -> (32bit integer=w653:i32)
            n571 = To Long Integer(number=w651) -> (32bit integer=w654:i32)
            n572 = Bundle(w656, w655) -> (w645:cluster{i32, i32})  [unwired: 1 in]
            n573 = Bundle(w653, w654) -> (w644:cluster{i32, i32})  [unwired: 1 in]
            n574 = property on="P1 Top Right Marker" class="Pict"("Position"=w645) -> ()  [unwired: 2 in, 2 out]
            n575 = property on="P1 Top Left Marker" class="Pict"("Position"=w644) -> ()  [unwired: 2 in, 2 out]
          }
        }
      }
      event "P2 Piece", "P2 Piece 2", "P2 Piece 3", "P2 Piece 4", "P2 Piece 5", "P2 Piece 6", "P2 Piece 7", "P2 Piece 8", "P2 Piece 9", "P2 Piece 10", "P2 Piece 11", "P2 Piece 12": Mouse Down {
        n576 = event-data() -> ("CtlRef"=w675:refnum<vi>)  [unwired: 1 in, 7 out]
        n577 = local read "P2 Turn Light"() -> (w676:bool)
        n578 = case shown="True" w676 {
          tunnel: w675 -> [_ w679]
          frame False {
            # "It's not player 1's turn yet. Do nothing."
          }
          frame True {
            # "This sub VI outputs a 2d array \nthat holds 2 coordinates indicating \nwhere the piece can go"
            # "At this point, I use an \nequation to turn the pixel\ncoordinates into the array coordinates\nof the piece that the user clicked."
            # "Left first"
            # "row[0], collumn[1]"
            n579 = property on="Property Node" class="Pict"(reference=w679) -> ("Position"=w680:T1)  [unwired: 1 in, 2 out]
            n580 = global read "Board Layout Global Variable.vi" "Board Layout"() -> (w709:dbl[][])
            n581 = Unbundle By Name(w680) -> ("Left"=w698:i32, "Top"=w696:i32)
            n582 = expression code="(x-469)/42"(w698) -> (w699:i32)
            n583 = expression code="(x-56)/42"(w696) -> (w697:i32)
            n584 = To Long Integer(number=w699) -> (32bit integer=w681:i32)
            n585 = To Long Integer(number=w697) -> (32bit integer=w682:i32)
            n586 = Build Array(w682, w681) -> (w708:i32[])
            n587 = call "MoveLogic.vi"("Coordinates"=w708, "Array"=w709) -> ("Moves"=w705:dbl[][])
            n588 = Index Array(array=w705, index (row)=0) -> (element=w683:dbl[])  [unwired: 1 in]
            n589 = Index Array(array=w705, index (row)=1) -> (element=w702:dbl[])  [unwired: 1 in]
            n590 = Index Array(array=w702, index=1) -> (element=w695:dbl)
            n591 = Index Array(array=w702, index=0) -> (element=w694:dbl)
            n592 = Index Array(array=w683, index=0) -> (element=w684:dbl)
            n593 = Index Array(array=w683, index=1) -> (element=w685:dbl)
            n594 = expression code="(x*42)+56"(w694) -> (w693:dbl)
            n595 = expression code="(x*42)+469"(w695) -> (w692:dbl)
            n596 = expression code="(x*42)+56"(w684) -> (w686:dbl)
            n597 = expression code="(x*42)+469"(w685) -> (w687:dbl)
            n598 = To Long Integer(number=w692) -> (32bit integer=w691:i32)
            n599 = To Long Integer(number=w693) -> (32bit integer=w690:i32)
            n600 = To Long Integer(number=w687) -> (32bit integer=w688:i32)
            n601 = To Long Integer(number=w686) -> (32bit integer=w689:i32)
            n602 = Bundle(w691, w690) -> (w678:cluster{i32, i32})  [unwired: 1 in]
            n603 = Bundle(w688, w689) -> (w677:cluster{i32, i32})  [unwired: 1 in]
            n604 = property on="P2 Bottom Left Marker" class="Pict"("Position"=w677) -> ()  [unwired: 2 in, 2 out]
            n605 = property on="P2 Bottom Right Marker" class="Pict"("Position"=w678) -> ()  [unwired: 2 in, 2 out]
          }
        }
      }
      event "P2 King", "P2 King 2", "P2 King 3", "P2 King 4", "P2 King 5", "P2 King 6", "P2 King 7", "P2 King 8", "P2 King 9", "P2 King 10", "P2 King 11", "P2 King 12": Mouse Down {
        n606 = event-data() -> ("CtlRef"=w710:refnum<vi>)  [unwired: 1 in, 7 out]
        n607 = local read "P2 Turn Light"() -> (w711:bool)
        n608 = case shown="True" w711 {
          tunnel: w710 -> [_ w712]
          frame False {
            # "It's not player 1's turn yet. Do nothing."
          }
          frame True {
            # "At this point, I use an \nequation to turn the pixel\ncoordinates into the array coordinates\nof the piece that the user clicked."
            # "Left first"
            # "row[0], collumn[1]"
            n609 = property on="Property Node" class="Pict"(reference=w712) -> ("Position"=w713:T1)  [unwired: 1 in, 2 out]
            n610 = global read "Board Layout Global Variable.vi" "Board Layout"() -> (w744:dbl[][])
            n611 = Unbundle By Name(w713) -> ("Left"=w733:i32, "Top"=w731:i32)
            n612 = expression code="(x-469)/42"(w733) -> (w734:i32)
            n613 = expression code="(x-56)/42"(w731) -> (w732:i32)
            n614 = To Long Integer(number=w734) -> (32bit integer=w716:i32)
            n615 = To Long Integer(number=w732) -> (32bit integer=w717:i32)
            n616 = Build Array(w717, w716) -> (w743:i32[])
            n617 = call "MoveLogic.vi"("Coordinates"=w743, "Array"=w744) -> ("Moves"=w740:dbl[][])
            n618 = Index Array(array=w740, index (row)=0) -> (element=w718:dbl[])  [unwired: 1 in]
            n619 = Index Array(array=w740, index (row)=1) -> (element=w737:dbl[])  [unwired: 1 in]
            n620 = Index Array(array=w737, index=1) -> (element=w730:dbl)
            n621 = Index Array(array=w737, index=0) -> (element=w729:dbl)
            n622 = Index Array(array=w718, index=0) -> (element=w719:dbl)
            n623 = Index Array(array=w718, index=1) -> (element=w720:dbl)
            n624 = expression code="(x*42)+56"(w729) -> (w728:dbl)
            n625 = expression code="(x*42)+469"(w730) -> (w727:dbl)
            n626 = expression code="(x*42)+56"(w719) -> (w721:dbl)
            n627 = expression code="(x*42)+469"(w720) -> (w722:dbl)
            n628 = To Long Integer(number=w727) -> (32bit integer=w726:i32)
            n629 = To Long Integer(number=w728) -> (32bit integer=w725:i32)
            n630 = To Long Integer(number=w722) -> (32bit integer=w723:i32)
            n631 = To Long Integer(number=w721) -> (32bit integer=w724:i32)
            n632 = Bundle(w726, w725) -> (w715:cluster{i32, i32})  [unwired: 1 in]
            n633 = Bundle(w723, w724) -> (w714:cluster{i32, i32})  [unwired: 1 in]
            n634 = property on="P1 Top Right Marker" class="Pict"("Position"=w715) -> ()  [unwired: 2 in, 2 out]
            n635 = property on="P1 Top Left Marker" class="Pict"("Position"=w714) -> ()  [unwired: 2 in, 2 out]
          }
        }
      }
      event "P1 Top Left Marker": Mouse Down {
        n636 = event-data() -> ()  [unwired: 1 in, 8 out]
        n637 = global read "Board Layout Global Variable.vi" "Board Layout"() -> (w746:dbl[][])
        n638 = property on="P1 Top Left Marker" class="Pict"() -> (error out=w752:errorcluster, "Position"=w754:T1)  [unwired: 2 in, 1 out]
        n639 = call "FixArray.vi"("PreviousState"=w746, "Cluster"=w747, "Array 3"=w748) -> ("NewState"=w745:dbl[][])
        n640 = global write "Board Layout Global Variable.vi" "Board Layout"(w745) -> ()
        n641 = property on="Property Node" class="Pict"(reference=w755, "Position"=w754) -> ()  [unwired: 1 in, 2 out]
        n642 = property on="P1 Bottom Left Marker" class="Pict"("Position"=T1 {"Left"=666, "Top"=666}) -> ()  [unwired: 2 in, 2 out]
        n643 = property on="P1 Bottom Right Marker" class="Pict"("Position"=T1 {"Left"=666, "Top"=666}) -> ()  [unwired: 2 in, 2 out]
        n644 = property on="P1 Top Left Marker" class="Pict"(error in=w752, "Position"=T1 {"Left"=666, "Top"=666}) -> ()  [unwired: 1 in, 2 out]
        n645 = property on="P1 Top Right Marker" class="Pict"("Position"=T1 {"Left"=666, "Top"=666}) -> ()  [unwired: 2 in, 2 out]
      }
      event "P2 Top Left Marker": Mouse Down {
        n646 = event-data() -> ()  [unwired: 1 in, 8 out]
        n647 = property on="P2 Top Left Marker" class="Pict"() -> (error out=w763:errorcluster, "Position"=w764:T1)  [unwired: 2 in, 1 out]
        n648 = local read "P1 Turn Light"() -> (w759:bool)
        n649 = property on="Property Node" class="Pict"(reference=w766, "Position"=w764) -> ()  [unwired: 1 in, 2 out]
        n650 = local read "P2 Turn Light"() -> (w757:bool)
        n651 = Not(x=w759) -> (.not. x?=w758:bool)
        n652 = Not(x=w757) -> (.not. x?=w756:bool)
        n653 = local write "P2 Turn Light"(w756) -> ()
        n654 = property on="P2 Bottom Right Marker" class="Pict"("Position"=T1 {"Left"=666, "Top"=666}) -> ()  [unwired: 2 in, 2 out]
        n655 = property on="P2 Top Left Marker" class="Pict"(error in=w763, "Position"=T1 {"Left"=666, "Top"=666}) -> ()  [unwired: 1 in, 2 out]
        n656 = property on="P2 Top Right Marker" class="Pict"("Position"=T1 {"Left"=666, "Top"=666}) -> ()  [unwired: 2 in, 2 out]
        n657 = local write "P1 Turn Light"(w758) -> ()
        n658 = property on="P2 Bottom Left Marker" class="Pict"("Position"=T1 {"Left"=666, "Top"=666}) -> ()  [unwired: 2 in, 2 out]
      }
      event "P2 Top Right Marker": Mouse Down {
        n659 = event-data() -> ()  [unwired: 1 in, 8 out]
        n660 = property on="P2 Top Right Marker" class="Pict"() -> (error out=w771:errorcluster, "Position"=w772:T1)  [unwired: 2 in, 1 out]
        n661 = local read "P1 Turn Light"() -> (w770:bool)
        n662 = local read "P2 Turn Light"() -> (w768:bool)
        n663 = property on="Property Node" class="Pict"(reference=w777, "Position"=w772) -> ()  [unwired: 1 in, 2 out]
        n664 = Not(x=w770) -> (.not. x?=w769:bool)
        n665 = Not(x=w768) -> (.not. x?=w767:bool)
        n666 = local write "P2 Turn Light"(w767) -> ()
        n667 = local write "P1 Turn Light"(w769) -> ()
        n668 = property on="P2 Bottom Right Marker" class="Pict"("Position"=T1 {"Left"=666, "Top"=666}) -> ()  [unwired: 2 in, 2 out]
        n669 = property on="P2 Top Left Marker" class="Pict"("Position"=T1 {"Left"=666, "Top"=666}) -> ()  [unwired: 2 in, 2 out]
        n670 = property on="P2 Top Right Marker" class="Pict"(error in=w771, "Position"=T1 {"Left"=666, "Top"=666}) -> ()  [unwired: 1 in, 2 out]
        n671 = property on="P2 Bottom Left Marker" class="Pict"("Position"=T1 {"Left"=666, "Top"=666}) -> ()  [unwired: 2 in, 2 out]
      }
      event "P2 Bottom Left Marker": Mouse Down {
        n672 = event-data() -> ()  [unwired: 1 in, 8 out]
        n673 = property on="P2 Bottom Left Marker" class="Pict"() -> (error out=w782:errorcluster, "Position"=w783:T1)  [unwired: 2 in, 1 out]
        n674 = local read "P1 Turn Light"() -> (w781:bool)
        n675 = local read "P2 Turn Light"() -> (w779:bool)
        n676 = property on="Property Node" class="Pict"(reference=w788, "Position"=w783) -> ()  [unwired: 1 in, 2 out]
        n677 = Not(x=w781) -> (.not. x?=w780:bool)
        n678 = Not(x=w779) -> (.not. x?=w778:bool)
        n679 = local write "P2 Turn Light"(w778) -> ()
        n680 = local write "P1 Turn Light"(w780) -> ()
        n681 = property on="P2 Bottom Right Marker" class="Pict"("Position"=T1 {"Left"=666, "Top"=666}) -> ()  [unwired: 2 in, 2 out]
        n682 = property on="P2 Top Left Marker" class="Pict"("Position"=T1 {"Left"=666, "Top"=666}) -> ()  [unwired: 2 in, 2 out]
        n683 = property on="P2 Top Right Marker" class="Pict"("Position"=T1 {"Left"=666, "Top"=666}) -> ()  [unwired: 2 in, 2 out]
        n684 = property on="P2 Bottom Left Marker" class="Pict"(error in=w782, "Position"=T1 {"Left"=666, "Top"=666}) -> ()  [unwired: 1 in, 2 out]
      }
      event "P2 Bottom Right Marker": Mouse Down {
        n685 = event-data() -> ()  [unwired: 1 in, 8 out]
        n686 = property on="P2 Bottom Right Marker" class="Pict"() -> (error out=w793:errorcluster, "Position"=w794:T1)  [unwired: 2 in, 1 out]
        n687 = local read "P1 Turn Light"() -> (w792:bool)
        n688 = property on="Property Node" class="Pict"(reference=w799, "Position"=w794) -> ()  [unwired: 1 in, 2 out]
        n689 = local read "P2 Turn Light"() -> (w790:bool)
        n690 = Not(x=w792) -> (.not. x?=w791:bool)
        n691 = Not(x=w790) -> (.not. x?=w789:bool)
        n692 = local write "P2 Turn Light"(w789) -> ()
        n693 = property on="P2 Bottom Right Marker" class="Pict"(error in=w793, "Position"=T1 {"Left"=666, "Top"=666}) -> ()  [unwired: 1 in, 2 out]
        n694 = property on="P2 Top Left Marker" class="Pict"("Position"=T1 {"Left"=666, "Top"=666}) -> ()  [unwired: 2 in, 2 out]
        n695 = property on="P2 Top Right Marker" class="Pict"("Position"=T1 {"Left"=666, "Top"=666}) -> ()  [unwired: 2 in, 2 out]
        n696 = property on="P2 Bottom Left Marker" class="Pict"("Position"=T1 {"Left"=666, "Top"=666}) -> ()  [unwired: 2 in, 2 out]
        n697 = local write "P1 Turn Light"(w791) -> ()
      }
      event "P1 Top Right Marker": Mouse Down {
        n698 = event-data() -> ()  [unwired: 1 in, 8 out]
        n699 = property on="P1 Top Right Marker" class="Pict"() -> ("Position"=w809:T1)  [unwired: 2 in, 2 out]
        n700 = global read "Board Layout Global Variable.vi" "Board Layout"() -> (w803:dbl[][])
        n701 = call "FixArray.vi"("PreviousState"=w803, "Cluster"=w801, "Array 3"=w800) -> ("NewState"=w802:dbl[][])
        n702 = global write "Board Layout Global Variable.vi" "Board Layout"(w802) -> ()
        n703 = property on="Property Node" class="Pict"(reference=w814, "Position"=w809) -> (error out=w808:errorcluster)  [unwired: 1 in, 1 out]
        n704 = property on="P1 Bottom Left Marker" class="Pict"("Position"=T1 {"Left"=666, "Top"=666}) -> ()  [unwired: 2 in, 2 out]
        n705 = property on="P1 Bottom Right Marker" class="Pict"("Position"=T1 {"Left"=666, "Top"=666}) -> ()  [unwired: 2 in, 2 out]
        n706 = property on="P1 Top Left Marker" class="Pict"("Position"=T1 {"Left"=666, "Top"=666}) -> ()  [unwired: 2 in, 2 out]
        n707 = property on="P1 Top Right Marker" class="Pict"(error in=w808, "Position"=T1 {"Left"=666, "Top"=666}) -> ()  [unwired: 1 in, 2 out]
        n708 = local read "P1 Turn Light"() -> (w807:bool)
        n709 = local read "P2 Turn Light"() -> (w805:bool)
        n710 = Not(x=w807) -> (.not. x?=w806:bool)
        n711 = Not(x=w805) -> (.not. x?=w804:bool)
        n712 = local write "P2 Turn Light"(w804) -> ()
        n713 = local write "P1 Turn Light"(w806) -> ()
      }
      event "P1 Bottom Left Marker": Mouse Down {
        n714 = event-data() -> ()  [unwired: 1 in, 8 out]
        n715 = property on="P1 Bottom Left Marker" class="Pict"() -> ("Position"=w844:T1)  [unwired: 2 in, 2 out]
        n716 = local read "P1 Turn Light"() -> (w839:bool)
        n717 = local read "P1 Turn Light"() -> (w838:bool)
        n718 = local read "P1 Turn Light"() -> (w831:bool)
        n719 = local read "P1 Turn Light"() -> (w827:bool)
        n720 = local read "P1 Turn Light"() -> (w823:bool)
        n721 = local read "P1 Turn Light"() -> (w819:bool)
        n722 = local read "P1 Turn Light"() -> (w818:bool)
        n723 = local read "P2 Turn Light"() -> (w841:bool)
        n724 = local read "P2 Turn Light"() -> (w836:bool)
        n725 = local read "P2 Turn Light"() -> (w833:bool)
        n726 = local read "P2 Turn Light"() -> (w829:bool)
        n727 = local read "P2 Turn Light"() -> (w825:bool)
        n728 = local read "P2 Turn Light"() -> (w821:bool)
        n729 = local read "P2 Turn Light"() -> (w816:bool)
        n730 = property on="Property Node" class="Pict"(reference=w849, "Position"=w844) -> (error out=w843:errorcluster)  [unwired: 1 in, 1 out]
        n731 = Not(x=w839) -> (.not. x?=w840:bool)
        n732 = Not(x=w838) -> (.not. x?=w837:bool)
        n733 = Not(x=w831) -> (.not. x?=w832:bool)
        n734 = Not(x=w827) -> (.not. x?=w828:bool)
        n735 = Not(x=w823) -> (.not. x?=w824:bool)
        n736 = Not(x=w819) -> (.not. x?=w820:bool)
        n737 = Not(x=w818) -> (.not. x?=w817:bool)
        n738 = Not(x=w841) -> (.not. x?=w842:bool)
        n739 = Not(x=w836) -> (.not. x?=w835:bool)
        n740 = Not(x=w833) -> (.not. x?=w834:bool)
        n741 = Not(x=w829) -> (.not. x?=w830:bool)
        n742 = Not(x=w825) -> (.not. x?=w826:bool)
        n743 = Not(x=w821) -> (.not. x?=w822:bool)
        n744 = Not(x=w816) -> (.not. x?=w815:bool)
        n745 = local write "P2 Turn Light"(w842) -> ()
        n746 = local write "P2 Turn Light"(w835) -> ()
        n747 = local write "P2 Turn Light"(w834) -> ()
        n748 = local write "P2 Turn Light"(w830) -> ()
        n749 = local write "P2 Turn Light"(w826) -> ()
        n750 = local write "P2 Turn Light"(w822) -> ()
        n751 = local write "P2 Turn Light"(w815) -> ()
        n752 = local write "P1 Turn Light"(w840) -> ()
        n753 = local write "P1 Turn Light"(w837) -> ()
        n754 = local write "P1 Turn Light"(w832) -> ()
        n755 = local write "P1 Turn Light"(w828) -> ()
        n756 = local write "P1 Turn Light"(w824) -> ()
        n757 = local write "P1 Turn Light"(w820) -> ()
        n758 = local write "P1 Turn Light"(w817) -> ()
        n759 = property on="P1 Bottom Left Marker" class="Pict"(error in=w843, "Position"=T1 {"Left"=666, "Top"=666}) -> ()  [unwired: 1 in, 2 out]
        n760 = property on="P1 Bottom Right Marker" class="Pict"("Position"=T1 {"Left"=666, "Top"=666}) -> ()  [unwired: 2 in, 2 out]
        n761 = property on="P1 Top Left Marker" class="Pict"("Position"=T1 {"Left"=666, "Top"=666}) -> ()  [unwired: 2 in, 2 out]
        n762 = property on="P1 Top Right Marker" class="Pict"("Position"=T1 {"Left"=666, "Top"=666}) -> ()  [unwired: 2 in, 2 out]
      }
      event "P1 Bottom Right Marker": Mouse Down {
        n763 = event-data() -> ()  [unwired: 1 in, 8 out]
        n764 = property on="P1 Bottom Right Marker" class="Pict"() -> ("Position"=w935:T1)  [unwired: 2 in, 2 out]
        n765 = local read "P1 Turn Light"() -> (w930:bool)
        n766 = local read "P1 Turn Light"() -> (w929:bool)
        n767 = local read "P1 Turn Light"() -> (w922:bool)
        n768 = local read "P1 Turn Light"() -> (w918:bool)
        n769 = local read "P1 Turn Light"() -> (w914:bool)
        n770 = local read "P1 Turn Light"() -> (w910:bool)
        n771 = local read "P1 Turn Light"() -> (w909:bool)
        n772 = local read "P1 Turn Light"() -> (w881:bool)
        n773 = local read "P1 Turn Light"() -> (w882:bool)
        n774 = local read "P1 Turn Light"() -> (w889:bool)
        n775 = local read "P1 Turn Light"() -> (w893:bool)
        n776 = local read "P1 Turn Light"() -> (w897:bool)
        n777 = local read "P1 Turn Light"() -> (w901:bool)
        n778 = local read "P1 Turn Light"() -> (w902:bool)
        n779 = local read "P1 Turn Light"() -> (w874:bool)
        n780 = local read "P1 Turn Light"() -> (w873:bool)
        n781 = local read "P1 Turn Light"() -> (w866:bool)
        n782 = local read "P1 Turn Light"() -> (w862:bool)
        n783 = local read "P1 Turn Light"() -> (w858:bool)
        n784 = local read "P1 Turn Light"() -> (w854:bool)
        n785 = local read "P1 Turn Light"() -> (w853:bool)
        n786 = local read "P2 Turn Light"() -> (w932:bool)
        n787 = local read "P2 Turn Light"() -> (w927:bool)
        n788 = local read "P2 Turn Light"() -> (w924:bool)
        n789 = local read "P2 Turn Light"() -> (w920:bool)
        n790 = local read "P2 Turn Light"() -> (w916:bool)
        n791 = local read "P2 Turn Light"() -> (w912:bool)
        n792 = local read "P2 Turn Light"() -> (w907:bool)
        n793 = local read "P2 Turn Light"() -> (w879:bool)
        n794 = local read "P2 Turn Light"() -> (w884:bool)
        n795 = local read "P2 Turn Light"() -> (w887:bool)
        n796 = local read "P2 Turn Light"() -> (w891:bool)
        n797 = local read "P2 Turn Light"() -> (w895:bool)
        n798 = local read "P2 Turn Light"() -> (w899:bool)
        n799 = local read "P2 Turn Light"() -> (w904:bool)
        n800 = local read "P2 Turn Light"() -> (w876:bool)
        n801 = local read "P2 Turn Light"() -> (w871:bool)
        n802 = local read "P2 Turn Light"() -> (w868:bool)
        n803 = local read "P2 Turn Light"() -> (w864:bool)
        n804 = local read "P2 Turn Light"() -> (w860:bool)
        n805 = local read "P2 Turn Light"() -> (w856:bool)
        n806 = local read "P2 Turn Light"() -> (w851:bool)
        n807 = property on="Property Node" class="Pict"(reference=w940, "Position"=w935) -> (error out=w934:errorcluster)  [unwired: 1 in, 1 out]
        n808 = Not(x=w930) -> (.not. x?=w931:bool)
        n809 = Not(x=w929) -> (.not. x?=w928:bool)
        n810 = Not(x=w922) -> (.not. x?=w923:bool)
        n811 = Not(x=w918) -> (.not. x?=w919:bool)
        n812 = Not(x=w914) -> (.not. x?=w915:bool)
        n813 = Not(x=w910) -> (.not. x?=w911:bool)
        n814 = Not(x=w909) -> (.not. x?=w908:bool)
        n815 = Not(x=w881) -> (.not. x?=w880:bool)
        n816 = Not(x=w882) -> (.not. x?=w883:bool)
        n817 = Not(x=w889) -> (.not. x?=w888:bool)
        n818 = Not(x=w893) -> (.not. x?=w892:bool)
        n819 = Not(x=w897) -> (.not. x?=w896:bool)
        n820 = Not(x=w901) -> (.not. x?=w900:bool)
        n821 = Not(x=w902) -> (.not. x?=w903:bool)
        n822 = Not(x=w874) -> (.not. x?=w875:bool)
        n823 = Not(x=w873) -> (.not. x?=w872:bool)
        n824 = Not(x=w866) -> (.not. x?=w867:bool)
        n825 = Not(x=w862) -> (.not. x?=w863:bool)
        n826 = Not(x=w858) -> (.not. x?=w859:bool)
        n827 = Not(x=w854) -> (.not. x?=w855:bool)
        n828 = Not(x=w853) -> (.not. x?=w852:bool)
        n829 = Not(x=w932) -> (.not. x?=w933:bool)
        n830 = Not(x=w927) -> (.not. x?=w926:bool)
        n831 = Not(x=w924) -> (.not. x?=w925:bool)
        n832 = Not(x=w920) -> (.not. x?=w921:bool)
        n833 = Not(x=w916) -> (.not. x?=w917:bool)
        n834 = Not(x=w912) -> (.not. x?=w913:bool)
        n835 = Not(x=w907) -> (.not. x?=w906:bool)
        n836 = Not(x=w879) -> (.not. x?=w878:bool)
        n837 = Not(x=w884) -> (.not. x?=w885:bool)
        n838 = Not(x=w887) -> (.not. x?=w886:bool)
        n839 = Not(x=w891) -> (.not. x?=w890:bool)
        n840 = Not(x=w895) -> (.not. x?=w894:bool)
        n841 = Not(x=w899) -> (.not. x?=w898:bool)
        n842 = Not(x=w904) -> (.not. x?=w905:bool)
        n843 = Not(x=w876) -> (.not. x?=w877:bool)
        n844 = Not(x=w871) -> (.not. x?=w870:bool)
        n845 = Not(x=w868) -> (.not. x?=w869:bool)
        n846 = Not(x=w864) -> (.not. x?=w865:bool)
        n847 = Not(x=w860) -> (.not. x?=w861:bool)
        n848 = Not(x=w856) -> (.not. x?=w857:bool)
        n849 = Not(x=w851) -> (.not. x?=w850:bool)
        n850 = local write "P2 Turn Light"(w933) -> ()
        n851 = local write "P2 Turn Light"(w926) -> ()
        n852 = local write "P2 Turn Light"(w925) -> ()
        n853 = local write "P2 Turn Light"(w921) -> ()
        n854 = local write "P2 Turn Light"(w917) -> ()
        n855 = local write "P2 Turn Light"(w913) -> ()
        n856 = local write "P2 Turn Light"(w906) -> ()
        n857 = local write "P2 Turn Light"(w878) -> ()
        n858 = local write "P2 Turn Light"(w885) -> ()
        n859 = local write "P2 Turn Light"(w886) -> ()
        n860 = local write "P2 Turn Light"(w890) -> ()
        n861 = local write "P2 Turn Light"(w894) -> ()
        n862 = local write "P2 Turn Light"(w898) -> ()
        n863 = local write "P2 Turn Light"(w905) -> ()
        n864 = local write "P2 Turn Light"(w877) -> ()
        n865 = local write "P2 Turn Light"(w870) -> ()
        n866 = local write "P2 Turn Light"(w869) -> ()
        n867 = local write "P2 Turn Light"(w865) -> ()
        n868 = local write "P2 Turn Light"(w861) -> ()
        n869 = local write "P2 Turn Light"(w857) -> ()
        n870 = local write "P2 Turn Light"(w850) -> ()
        n871 = local write "P1 Turn Light"(w931) -> ()
        n872 = local write "P1 Turn Light"(w928) -> ()
        n873 = local write "P1 Turn Light"(w923) -> ()
        n874 = local write "P1 Turn Light"(w919) -> ()
        n875 = local write "P1 Turn Light"(w915) -> ()
        n876 = local write "P1 Turn Light"(w911) -> ()
        n877 = local write "P1 Turn Light"(w908) -> ()
        n878 = local write "P1 Turn Light"(w880) -> ()
        n879 = local write "P1 Turn Light"(w883) -> ()
        n880 = local write "P1 Turn Light"(w888) -> ()
        n881 = local write "P1 Turn Light"(w892) -> ()
        n882 = local write "P1 Turn Light"(w896) -> ()
        n883 = local write "P1 Turn Light"(w900) -> ()
        n884 = local write "P1 Turn Light"(w903) -> ()
        n885 = local write "P1 Turn Light"(w875) -> ()
        n886 = local write "P1 Turn Light"(w872) -> ()
        n887 = local write "P1 Turn Light"(w867) -> ()
        n888 = local write "P1 Turn Light"(w863) -> ()
        n889 = local write "P1 Turn Light"(w859) -> ()
        n890 = local write "P1 Turn Light"(w855) -> ()
        n891 = local write "P1 Turn Light"(w852) -> ()
        n892 = property on="P1 Top Left Marker" class="Pict"("Position"=T1 {"Left"=666, "Top"=666}) -> ()  [unwired: 2 in, 2 out]
        n893 = property on="P1 Top Right Marker" class="Pict"("Position"=T1 {"Left"=666, "Top"=666}) -> ()  [unwired: 2 in, 2 out]
        n894 = property on="P1 Bottom Right Marker" class="Pict"(error in=w934, "Position"=T1 {"Left"=666, "Top"=666}) -> ()  [unwired: 1 in, 2 out]
        n895 = property on="P1 Bottom Left Marker" class="Pict"("Position"=T1 {"Left"=666, "Top"=666}) -> ()  [unwired: 2 in, 2 out]
      }
    }
  }
  n896 = stacked-sequence {
    frame #0 {
      n897 = call "Checkers P1 Turn Drawer.vi"() -> ("new picture"=→"P1 Top Right Marker":picture)  [unwired: 11 in]
      n898 = property on="P1 Top Right Marker" class="Pict"("Position"=T1 {"Left"=666, "Top"=666}) -> ()  [unwired: 2 in, 2 out]
    }
    frame #1 {
      n899 = call "Checkers P1 Turn Drawer.vi"() -> ("new picture"=→"P1 Top Left Marker":picture)  [unwired: 11 in]
      n900 = property on="P1 Top Left Marker" class="Pict"("Position"=T1 {"Left"=666, "Top"=666}) -> ()  [unwired: 2 in, 2 out]
    }
    frame #2 {
      n901 = call "Checkers P1 Turn Drawer.vi"() -> ("new picture"=→"P1 Bottom Left Marker":picture)  [unwired: 11 in]
      n902 = property on="P1 Bottom Left Marker" class="Pict"("Position"=T1 {"Left"=666, "Top"=666}) -> ()  [unwired: 2 in, 2 out]
    }
    frame #3 {
      n903 = call "Checkers P1 Turn Drawer.vi"() -> ("new picture"=→"P1 Bottom Right Marker":picture)  [unwired: 11 in]
      n904 = property on="P1 Bottom Right Marker" class="Pict"("Position"=T1 {"Left"=666, "Top"=666}) -> ()  [unwired: 2 in, 2 out]
    }
    frame #4 {
      n905 = call "Checkers P2 Turn Drawer.vi"() -> ("new picture"=→"P2 Top Left Marker":picture)  [unwired: 11 in]
      n906 = property on="P2 Top Left Marker" class="Pict"("Position"=T1 {"Left"=666, "Top"=666}) -> ()  [unwired: 2 in, 2 out]
    }
    frame #5 {
      n907 = call "Checkers P2 Turn Drawer.vi"() -> ("new picture"=→"P2 Top Right Marker":picture)  [unwired: 11 in]
      n908 = property on="P2 Top Right Marker" class="Pict"("Position"=T1 {"Left"=666, "Top"=666}) -> ()  [unwired: 2 in, 2 out]
    }
    frame #6 {
      n909 = call "Checkers P2 Turn Drawer.vi"() -> ("new picture"=→"P2 Bottom Left Marker":picture)  [unwired: 11 in]
      n910 = property on="P2 Bottom Left Marker" class="Pict"("Position"=T1 {"Left"=666, "Top"=666}) -> ()  [unwired: 2 in, 2 out]
    }
    frame #7 {
      n911 = call "Checkers P2 Turn Drawer.vi"() -> ("new picture"=→"P2 Bottom Right Marker":picture)  [unwired: 11 in]
      n912 = property on="P2 Bottom Right Marker" class="Pict"("Position"=T1 {"Left"=666, "Top"=666}) -> ()  [unwired: 2 in, 2 out]
    }
  }
  "Player 1 Label" <- "Player 1" ("String 3")
  "Player 2 Label" <- "Player 2" ("String 4")
